vi "main_grid_forming.vi"() -> ()   [LabVIEW 2021]
uses:
  <vilib>/xnet/xnet.llb/XNET Frame CAN.ctl
  <vilib>/xnet/xnet.llb/XNET Frame Type CAN.ctl
  Helper functions/General Purpose/references.ctl
  Helper functions/General Purpose/measurements.ctl
  Helper functions/Time-sync/time_sync/TypeDef/Synch_shift--cluster.ctl
  <vilib>/Platform/TimedLoop/XDataNode/timing_clust.ctl
  <vilib>/Platform/TimedLoop/XDataNode/nitl_modes.ctl
  <vilib>/Platform/TimedLoop/XDataNode/wakeup.ctl
  Helper functions/communication/AFE_froming_Central.ctl
  Helper functions/communication/AFE_froming_Central_Info.ctl
  Helper functions/communication/AFE_froming_Central_Data.ctl
  <vilib>/xnet/xnet.llb/XNET Write (Frame CAN).vi
  <vilib>/xnet/xnet.llb/XNET Read (Frame CAN).vi
  <vilib>/Platform/TimedLoop/XDataNode/XDataNode.xnode
  <vilib>/Platform/TimedLoop/XDataNode/XDNodeRunTimeDep.lvlib
  <userlib>/_OpenG.lib/boolean/boolean.llb/openg_boolean__ogtk.lvlib
panel:
  in  "delta V":dbl format="%#_13g"
  in  "delta f":dbl=0.005800000000000027 format="%#_13g"
  in  "biasQ4":dbl=200.0
  in  "biasQ3":dbl=200.0
  in  "biasQ2":dbl=200.0
  in  "biasQ1":dbl=200.0
  in  "biasV4":dbl
  in  "biasV3":dbl
  in  "biasV2":dbl
  in  "biasV1":dbl=0.6
  out "form":timestamp
  out "follow":timestamp
  out "time_afe":timestamp
  out "start following 1 pre":bool
  out "t_rising":timestamp
  out "t_risingedge":dbl
  out "Synch Monitor":string[][](table)
  in  "Loop Time":u32=125
  out "Error out":errorcluster
  in  "Timeout [ms]":i32=3000
  out "Offset from TR (ns)":dbl
  out "Status Out":T1
  out "CAN OUT":T2[](array[typedef]) {"payload" format="%x"; "timestamp" format="%<%.7X\n%x>T"; "type" items=["CAN Data"=0, "CAN Remote"=1, "CAN Bus Error"=2, "CAN 2.0 Data"=8, "CAN FD Data"=16, "CAN FD+BRS Data"=24, "J1939 Data"=192, "Delay"=224, "Log Trigger"=225, "Start Trigger"=226]; "identifier" format="%x"}
  in  "freq 2":dbl=50.0
  in  "freq 1":dbl=50.0
  in  "Vabs 1":dbl=230.0
  in  "Varg 1":dbl
  in  "Start following 2":bool
  in  "Start following 1":bool
  in  "Vabs 2":dbl=230.0
  in  "Varg 2":dbl
  out "Forming 2":bool
  out "Forming 1":bool
  in  "Start forming 2":bool
  in  "Start forming 1":bool
  out "current time":timestamp
  in  "measurements":T4
  in  "references":T5
  in  "To ACT CH 4":bool
  in  "To ACT CH 3":bool
  in  "To ACT CH 2":bool
  out "Error 4":bool
  out "Fault 4":bool
  out "Error 3":bool
  out "Fault 3":bool
  out "Error 2":bool
  out "Fault 2":bool
  out "State code 4":i32
  out "State code 3":i32
  out "State code 2":i32
  out "State code 1":i32
  out "Error 1":bool
  out "Fault 1":bool
  in  "To ACT CH 1":bool
  in  "main stop":bool
  in  "Vdc4":dbl=750.0
  in  "Qac4":dbl
  in  "Vdc3":dbl=750.0
  in  "Qac3":dbl
  in  "Vdc2":dbl=750.0
  in  "Qac2":dbl
  in  "Emergency 4":bool
  in  "To IN OP  4":bool
  in  "SEND sp 4":bool
  in  "Clear 4":bool
  in  "Shutdwn 4":bool
  in  "Emergency 3":bool
  in  "To IN OP  3":bool
  in  "SEND sp 3":bool
  in  "Clear 3":bool
  in  "Shutdwn 3":bool
  in  "Emergency 2":bool
  in  "To IN OP  2":bool
  in  "SEND sp 2":bool
  in  "Clear 2":bool
  in  "Shutdwn 2":bool
  out "V slider 22":dbl(slide) caption="V-i" max=-10.0 scale=650.0..780.0 scale format="%#_4g"
  out "V slider 21":dbl(slide) caption="V-i" max=-10.0 scale=650.0..780.0 scale format="%#_4g"
  out "V slider 20":dbl(slide) caption="V-i" max=-10.0 scale=650.0..780.0 scale format="%#_4g"
  out "kW":dbl caption="Numeric" format="%#.3g"
  out "?VkVAr":dbl caption="Numeric" format="%.3g"
  out "kW":dbl caption="Numeric" format="%#.3g"
  out "?VkVAr":dbl caption="Numeric" format="%.3g"
  out "kW":dbl caption="Numeric" format="%#.3g"
  out "?VkVAr":dbl caption="Numeric" format="%.3g"
  out "OFF 4":bool
  out "ON 4":bool
  out "Ready 4":bool
  out "OFF 3":bool
  out "ON 3":bool
  out "Ready 3":bool
  out "OFF 2":bool
  out "ON 2":bool
  out "Ready 2":bool
  out "error out":errorcluster
  out "?VkVAr":dbl caption="Numeric" format="%.3g"
  out "kW":dbl caption="Numeric" format="%#.3g"
  out "V slider 19":dbl(slide) caption="V-i" max=-10.0 scale=650.0..780.0 scale format="%#_4g"
  in  "Vdc1":dbl=750.0
  out "OFF 1":bool
  out "ON 1":bool
  out "Ready 1":bool
  out "CAN IN":T2 {"payload" format="%x"; "timestamp" format="%<%.7X\n%x>T"; "type" items=["CAN Data"=0, "CAN Remote"=1, "CAN Bus Error"=2, "CAN 2.0 Data"=8, "CAN FD Data"=16, "CAN FD+BRS Data"=24, "J1939 Data"=192, "Delay"=224, "Log Trigger"=225, "Start Trigger"=226]; "identifier" format="%x"}
  in  "Emergency 1":bool
  in  "Qac1":dbl
  in  "conv":T6
  in  "CAN [ms]":i64=1
  out "CAN with Conv":bool
  out "Measurements":bool
  in  "Shutdwn 1":bool
  in  "Clear 1":bool
  in  "SEND sp 1":bool
  in  "To IN OP 1":bool
  out "logging":bool
  # "Resource agents: AFE 1-4"
  # "package identifiers:\n1xx VSC1 \n2xx VSC2\n3xx VSC3\n4xx VSC4\n\nx0x send from agent to resource\nx02 Power setpoints\nx06 Measurements\nx9 status\n          = [state; error; alarm; OFF; Ready; ON]\n\n \n\nx1x send from resource to agent\nx10 Power measurements\nx11 Measurements\nx12 status\n          = [state; error; alarm; full; precharge; neg; 0; 0]"
  # "B18"
  # "B 22\nB19"
  # "VSC 4"
  # "B17"
  # "B21"
  # "VSC 3"
  # "B16"
  # "B20"
  # "Start-up - Shut down"
  # "VSC 2"
  # "B15"
  # "B19"
  # "Start-up - Shut down"
  # "VSC 1"
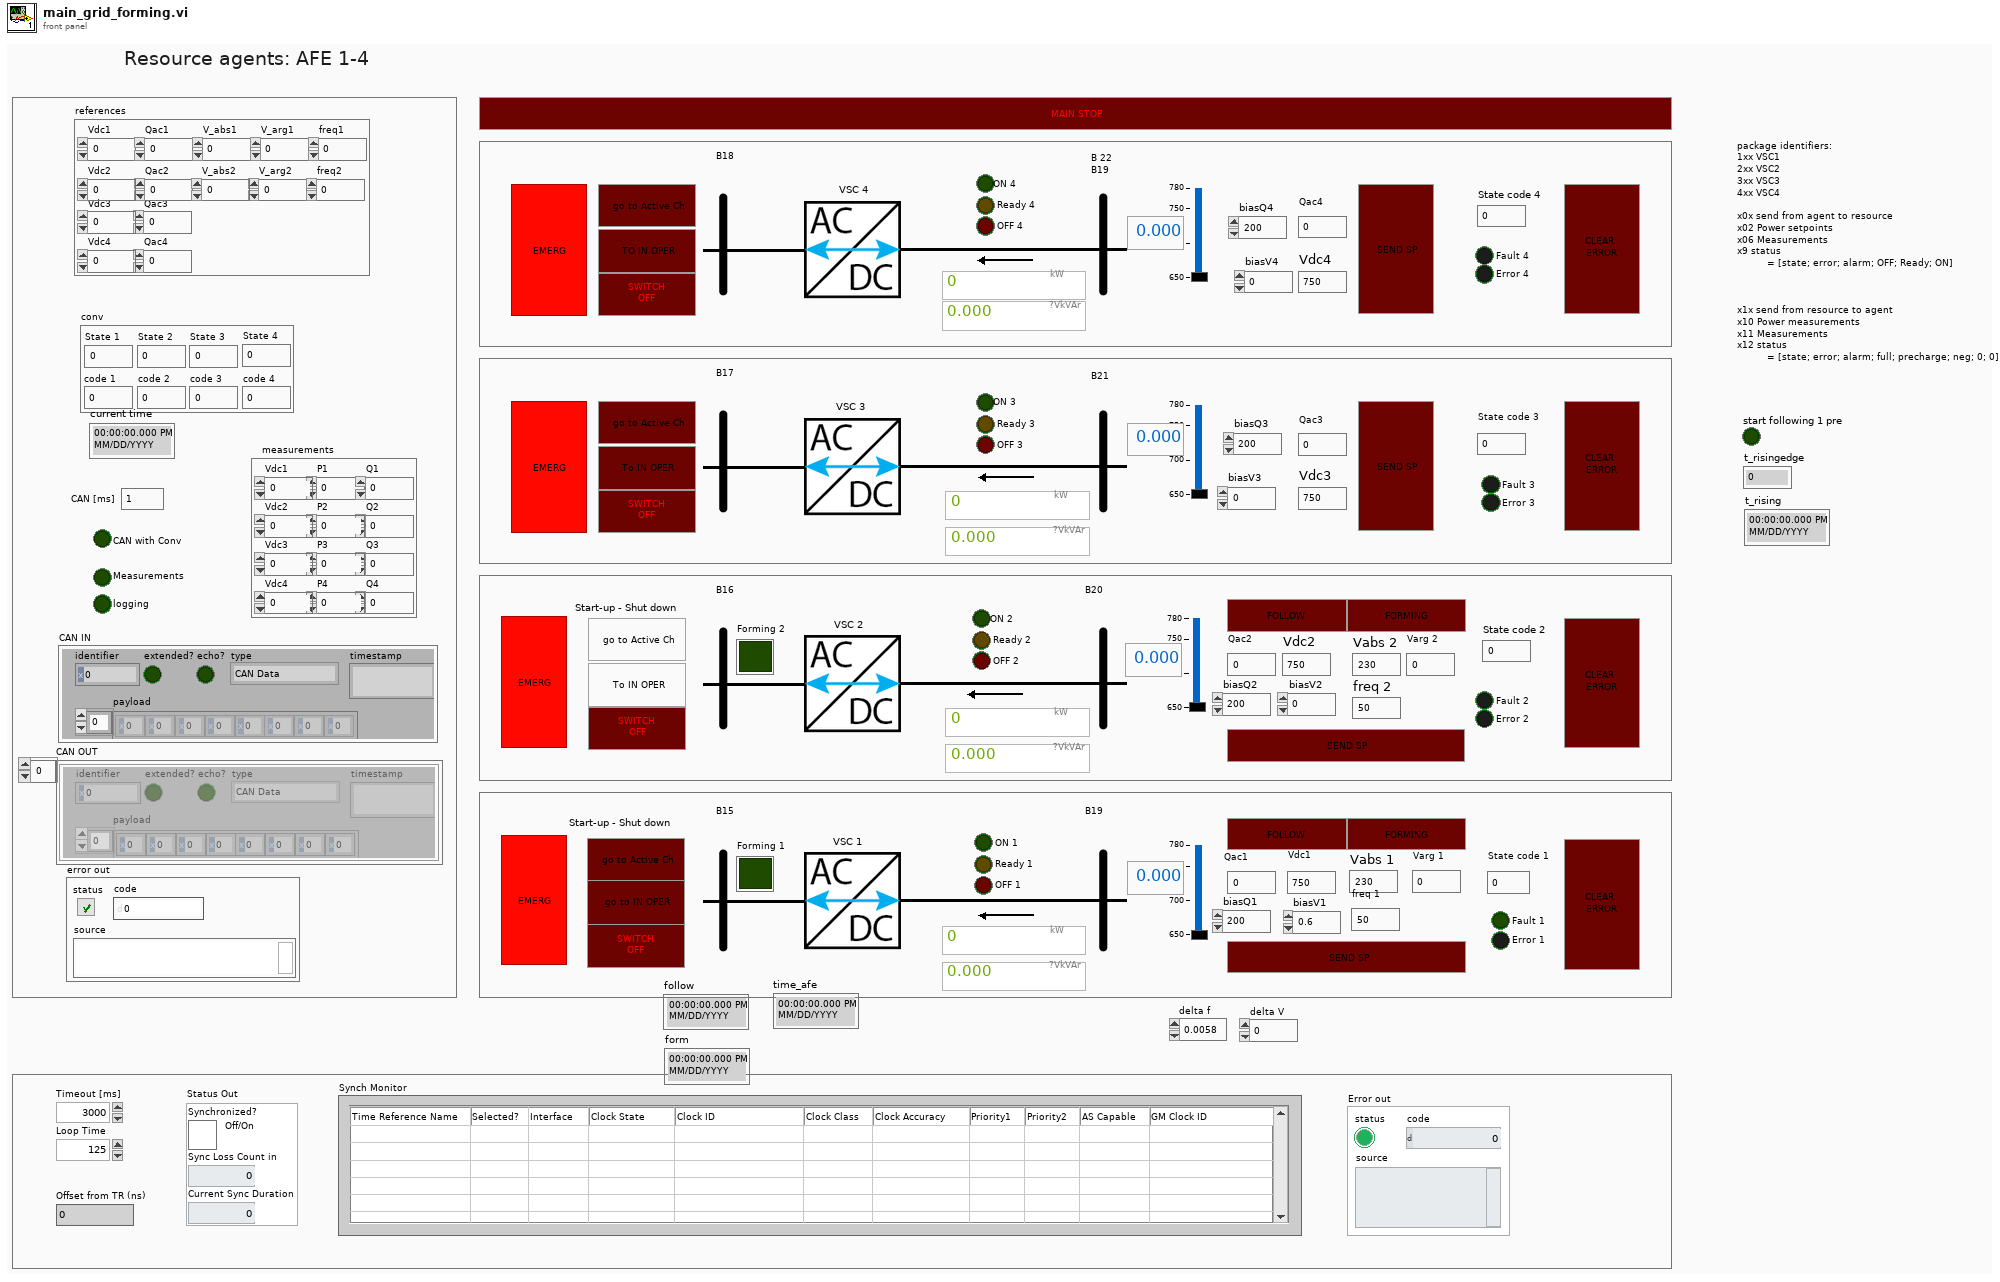
[diagram p1: front panel]
types:
  T1 = typedef "Synch_shift--cluster.ctl" = cluster{"Synchronized?":bool, "Sync Loss Count in":u32, "Current Sync Duration":u32}
  T2 = typedef "XNET Frame CAN.ctl" = cluster{"timestamp":timestamp, "payload":u8[], "identifier":u32, "type":T3, "extended?":bool, "echo?":bool}
  T3 = typedef "XNET Frame Type CAN.ctl" = u8
  T4 = typedef "measurements.ctl" = cluster{"Vdc1":dbl, "P1":dbl, "Vdc2":dbl, "P2":dbl, "Q2":dbl, "Vdc3":dbl, "P3":dbl, "Q3":dbl, "Vdc4":dbl, "P4":dbl, "Q4":dbl, "Q1":dbl}
  T5 = typedef "references.ctl" = cluster{"Vdc1":dbl, "Vdc2":dbl, "Qac2":dbl, "Vdc3":dbl, "Qac3":dbl, "Vdc4":dbl, "Qac4":dbl, "Qac1":dbl, "V_arg2":dbl, "V_abs2":dbl, "V_abs1":dbl, "V_arg1":dbl, "freq1":dbl, "freq2":dbl}
  T6 = cluster{"State 1":dbl, "code 1":dbl, "code 2":dbl, "code 3":dbl, "code 4":dbl, "State 2":dbl, "State 3":dbl, "State 4":dbl}
  T7 = cluster{"Frame In":refnum<k21>, "Frame Out":refnum<k21>}
  T8 = typedef "XDNodeRunTimeDep.lvlib/timing_clust.ctl" = cluster{"Expected End [f-1]":u64, "Actual End [f-1]":u64, "Finished Late? [f-1]":bool, "Expected End [i-1]":u64, "Actual End [i-1]":u64, "Finished Late? [i-1]":bool, "Expected Start [i]":u64, "Actual Start [i]":u64, "Expected Start [f]":u64, "Actual Start [f]":u64, "Source Name":string, "Structure Name":string, "Period":i64, "Deadline":i64, "Offset":i64, "Start":i64, "Priority":i32, "Timeout":i32, "Mode":T9, "Wakeup Reason":T10, "Error":errorcluster, "Source Type":string, "Secondary Source Type":string, "Global End Time":u64, "Global Start Time":u64, "Frame Duration":u64, "Iteration Duration":u64, "Assigned CPU":i32, "I/O Scan Engine Mode":u32}
  T9 = typedef "XDNodeRunTimeDep.lvlib/nitl_modes.ctl" = enum32{"No Change", "Process missed periods, maintain original phase", "Discard missed periods, maintain original phase", "Process missed periods, ignore original phase", "Discard missed periods, ignore original phase"}
  T10 = typedef "XDNodeRunTimeDep.lvlib/wakeup.ctl" = enum32{"Normal", "Aborted", "Asynchronous wakeup", "Timing source error", "Timed loop error", "Timeout"}
  T11 = typedef "AFE_froming_Central.ctl" = cluster{"Info":T12, "Data":T13}
  T12 = typedef "AFE_froming_Central_Info.ctl" = cluster{"Resource":string, "Problem":bool, "Timestamp":dbl}
  T13 = typedef "AFE_froming_Central_Data.ctl" = cluster{"Start forming 1":bool, "Forming/Following":bool[], "Start forming 2":bool, "measurements":cluster{"Vdc1":dbl, "P1":dbl, "Vdc2":dbl, "P2":dbl, "Q2":dbl, "Vdc3":dbl, "P3":dbl, "Q3":dbl, "Vdc4":dbl, "P4":dbl, "Q4":dbl, "Q1":dbl}, "Status":bool[], "references":T5, "Start following 1":bool, "Start following 2":bool}
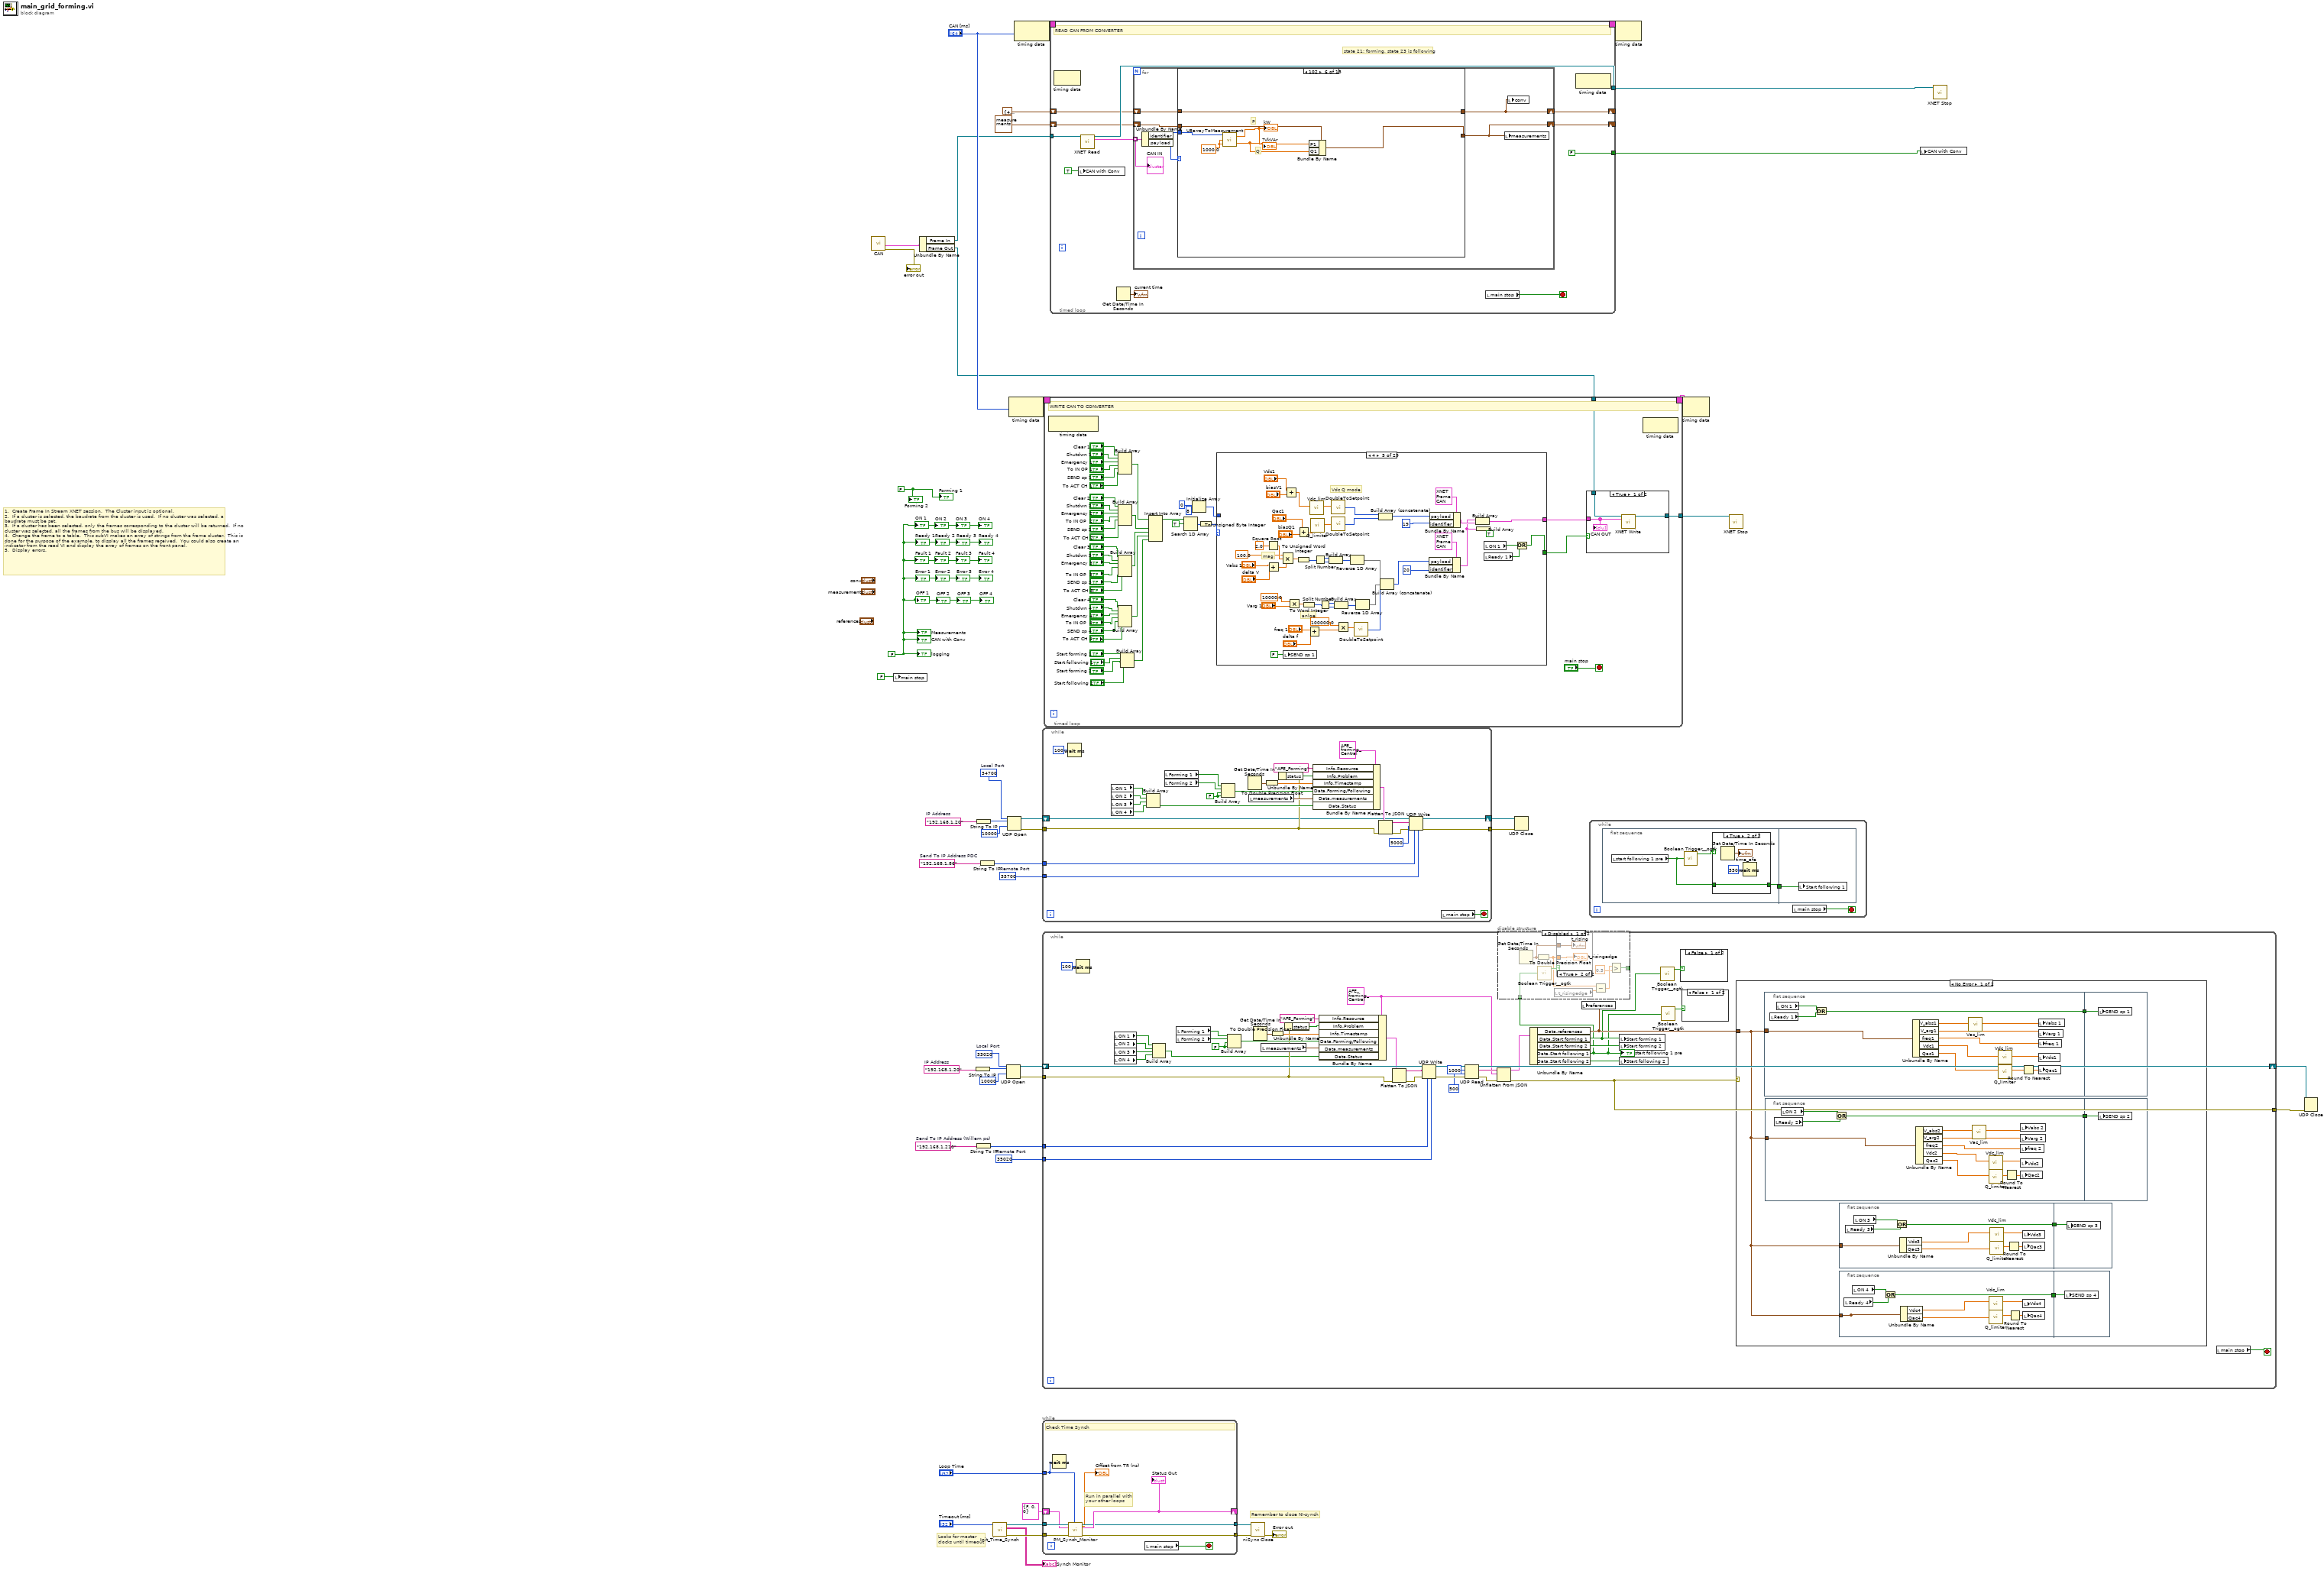
[diagram p0: block diagram]
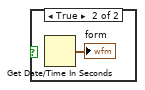
[diagram p3: hidden frame]
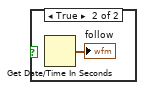
[diagram p4: hidden frame]
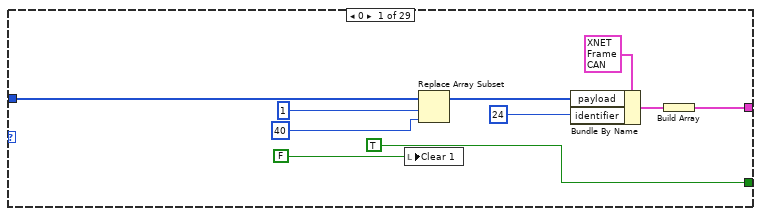
[diagram p9: hidden frame]
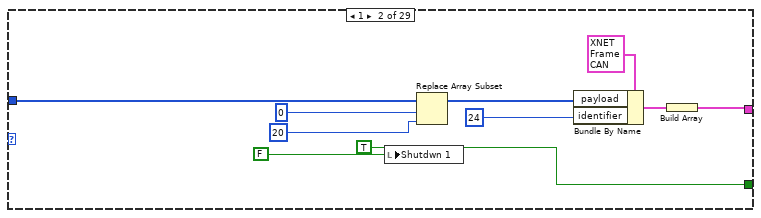
[diagram p10: hidden frame]
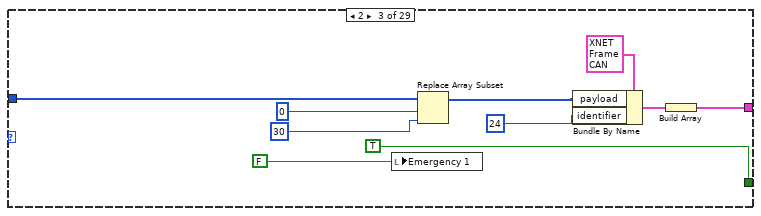
[diagram p11: hidden frame]
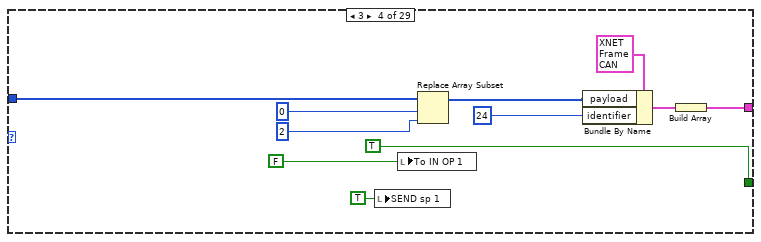
[diagram p12: hidden frame]
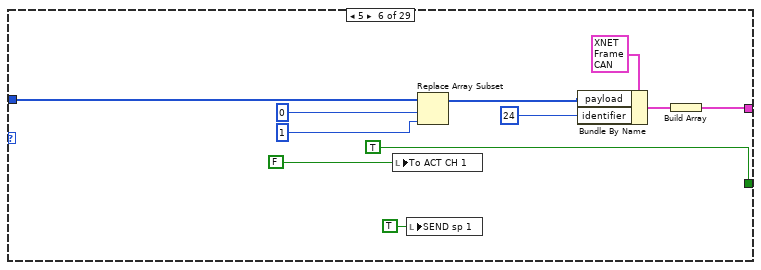
[diagram p13: hidden frame]
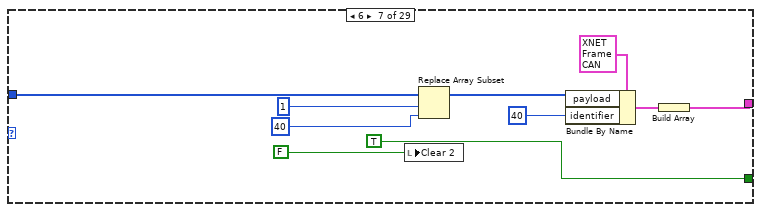
[diagram p14: hidden frame]
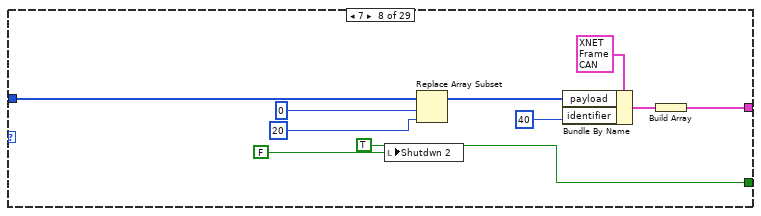
[diagram p15: hidden frame]
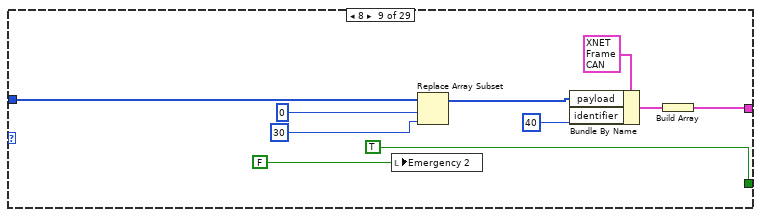
[diagram p16: hidden frame]
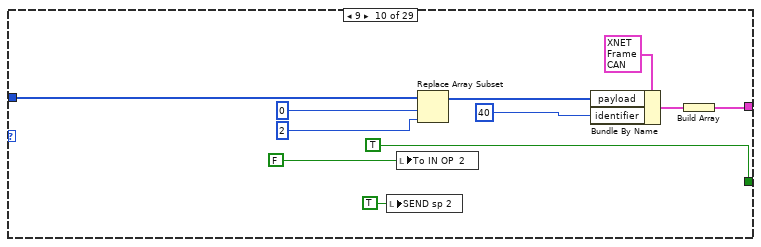
[diagram p17: hidden frame]
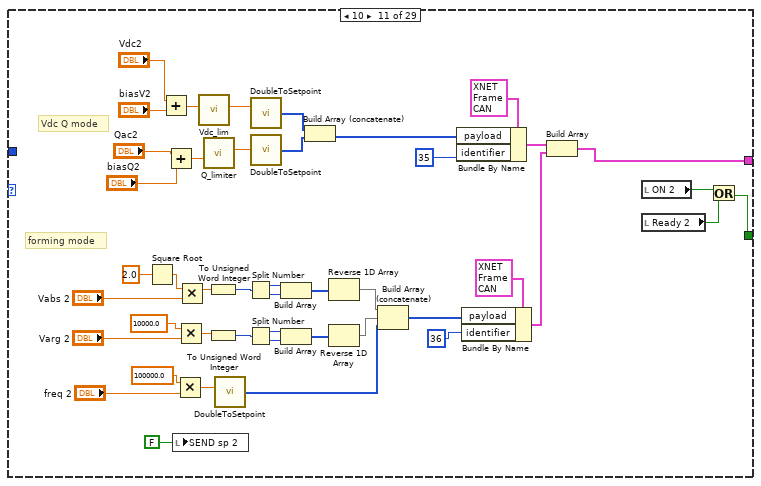
[diagram p18: hidden frame]
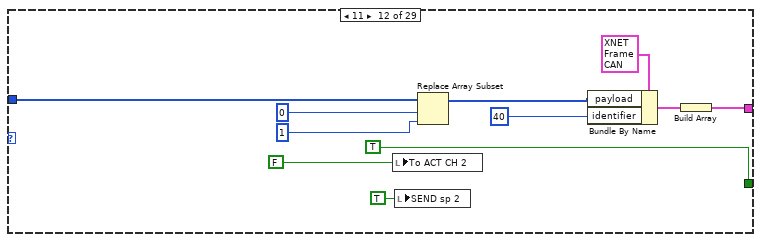
[diagram p19: hidden frame]
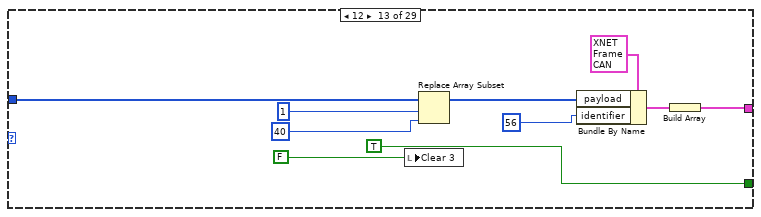
[diagram p20: hidden frame]
diagram:
  w7 = u16 35020  # Remote Port
  w13 = "192.168.1.210"  # Send To IP Address (Willem pc)
  w15 = u16 33020  # Local Port
  w16 = "192.168.1.20"  # IP Address
  w28 = FALSE ("Forming")
  w4 = u16 35700  # Remote Port
  w29 = "192.168.1.86"  # Send To IP Address PDC
  w31 = u16 34700  # Local Port
  w32 = "192.168.1.20"  # IP Address
  w34 = FALSE
  # "Remember to close NI-synch"
  # "Looks for master \nclocks until timeout"
  # "1.  Create Frame In Stream XNET session.  The Cluster input is optional.  \n2.  If a cluster is selected, the baudrate from the cluster is used.  If no cluster was selected, a baudrate must be set.\n3.  If a cluster has been selected, only the frames corresponding to the cluster will be returned.  If no cluster was selected, all the frames from the bus will be displayed.\n4.  Change the frame to a table.  This subVI makes an array of strings from the frame cluster.  This is done for the purpose of the example, to display all the frames received.  You could also create an indicator from the read VI and display the array of frames on the front panel. \n5.  Display errors."
  n1 = call "CAN.vi"() -> ("error out"=→"error out":errorcluster, "CAN"=w36:T7)  [unwired: 10 in]
  n2 = local write "main stop"(FALSE ("main stop")) -> ()
  n3 = Unbundle By Name(w36) -> ("Frame In"=w41:refnum<k21>, "Frame Out"=w44:refnum<k21>)
  n4 = String To IP(1:w16) -> (0:w17:u32)
  n5 = String To IP(1:w32) -> (0:w33:u32)
  n6 = String To IP(1:w13) -> (0:w8:u32)
  n7 = String To IP(1:w29) -> (0:w5:u32)
  n8 = call "Init_Time_Synch.vi"("Timeout [ms]"="Timeout [ms]") -> ("Error out"=w25:errorcluster, "Synch Monitor"=→"Synch Monitor":string[][], "Synch Out"=w23:refnum<k15>)  [unwired: 7 in, 1 out]
  n9 = UDP Open(7:w17, 9:10000 ("timeout ms (25000)"), 11:w15) -> (port=w12:refnum<k16>, 0:w11:errorcluster)  [unwired: 2 in, 1 out]
  n10 = UDP Open(7:w33, 9:10000 ("timeout ms (25000)"), 11:w31) -> (port=w3:refnum<k16>, 0:w2:errorcluster)  [unwired: 2 in, 1 out]
  n11 = node-c288("CAN [ms]") -> (w38:T8)
  n12 = node-c288("CAN [ms]") -> (w43:T8)
  n13 = while {
    tunnel: w11 -> [w66]
    shift-right: [w83] -> w10
    shift-left: w12 -> [w85]
    tunnel: [w86] -> w9
    tunnel: w8 -> [w75]
    tunnel: w7 -> [w79]
    stop <- w88 stop-if-true
    w63 = FALSE ("ON 1")
    w56 = T11 {"Info"={"Resource"="AFE_Forming", "Problem"=FALSE, "Timestamp"=0.0}, "Data"={"Start forming 1"=FALSE, "Forming/Following"=[], "Start forming 2"=FALSE, "measurements"={"Vdc1"=0.0, "P1"=0.0, "Vdc2"=0.0, "P2"=0.0, "Q2"=0.0, "Vdc3"=0.0, "P3"=0.0, "Q3"=0.0, "Vdc4"=0.0, "P4"=0.0, "Q4"=0.0, "Q1"=0.0}, "Status"=[], "references"={"Vdc1"=0.0, "Vdc2"=0.0, "Qac2"=0.0, "Vdc3"=0.0, "Qac3"=0.0, "Vdc4"=0.0, "Qac4"=0.0, "Qac1"=0.0, "V_arg2"=0.0, "V_abs2"=0.0, "V_abs1"=0.0, "V_arg1"=0.0, "freq1"=0.0, "freq2"=0.0}, "Start following 1"=FALSE, "Start following 2"=FALSE}} ("Cluster")
    n14 = Wait (ms)(milliseconds to wait=u32 100) -> ()  [unwired: 1 out]
    n15 = local read "ON 1"() -> (w61:bool)
    n16 = local read "ON 2"() -> (w62:bool)
    n17 = local read "ON 3"() -> (w59:bool)
    n18 = local read "ON 4"() -> (w58:bool)
    n19 = Build Array(w61, w62, w59, w58) -> (w60:bool[])
    n20 = local read "Forming 1"() -> (w65:bool)
    n21 = local read "Forming 2"() -> (w64:bool)
    n22 = Build Array(w65, w64, w63, w63) -> (w72:bool[])
    n23 = Get Date/Time In Seconds() -> (seconds since 1Jan1904=w68:timestamp)
    n24 = local read "measurements"() -> (w57:T4)
    n25 = To Double Precision Float(number=w68) -> (double precision float=w71:dbl)
    n26 = Unbundle By Name(w66) -> ("status"=w67:bool)
    n27 = Bundle By Name(cluster=w56, "Info.Resource"="AFE_Forming", "Info.Problem"=w67, "Info.Timestamp"=w71, "Data.Forming/Following"=w72, "Data.measurements"=w57, "Data.Status"=w60) -> (w69:T11)
    n28 = Flatten To JSON(anything=w69, error in (no error)=w66) -> (JSON string=w74:string, 11:w73:errorcluster)  [unwired: 1 in]
    n29 = UDP Write(address=w75, port or service name=w79, connection ID=w85, data in=w74, 8:w73) -> (error out=w81:errorcluster, 3:w84:refnum<k16>)  [unwired: 1 in]
    n30 = UDP Read(connection ID=w84, max size (548)=1000, timeout ms (25000)=500, 8:w81) -> (data out=w82:string, error out=w78:errorcluster, 3:w83:refnum<k16>)  [unwired: 2 out]
    n31 = Unflatten From JSON(JSON string=w82, type and defaults=w56, error in (no error)=w78) -> (value=w76:T11, error out=w86:errorcluster)  [unwired: 4 in]
    n32 = Unbundle By Name(w76) -> ("Data.references"=w87:T5, "Data.Start forming 1"=w50:bool, "Data.Start forming 2"=w54:bool, "Data.Start following 1"=w49:bool, "Data.Start following 2"=w53:bool)
    "start following 1 pre" <- w49
    n33 = disable-structure shown="Disabled" {
      disable-tunnel: [w95 _] -> _
      disable-tunnel: w49 -> [w93 _]
      frame Disabled {
        n34 = Get Date/Time In Seconds() -> (seconds since 1Jan1904=w94:timestamp)
        n35 = To Double Precision Float(number=w94) -> (double precision float=w96:dbl)
        n36 = call <userlib>:"Boolean Trigger__ogtk.vi"("Boolean Input"=w93) -> ("Rising Edge"=w98:bool)  [unwired: 1 in, 1 out]
        n37 = local read "t_risingedge"() -> (w97:dbl)
        n38 = case shown="True" w98 {
          tunnel: w96 -> [_ w100]
          tunnel: w94 -> [_ w99]
          frame False {
          }
          frame True {
            "t_risingedge" <- w100
            "t_rising" <- w99
          }
        }
        n39 = Subtract(x=w96, y=w97) -> (x-y=w92:dbl)
        n40 = Greater?(x=w92, y=0.5 ("x")) -> (0:w95:bool)
      }
      frame Enabled {
      }
    }
    n41 = local write "references"(w87) -> ()
    n42 = local write "Start forming 1"(w50) -> ()
    n43 = local write "Start forming 2"(w54) -> ()
    n44 = local write "Start following 2"(w53) -> ()
    n45 = call <userlib>:"Boolean Trigger__ogtk.vi"("Boolean Input"=w50) -> ("Rising Edge"=w51:bool)  [unwired: 1 in, 1 out]
    n46 = call <userlib>:"Boolean Trigger__ogtk.vi"("Boolean Input"=w49) -> ("Rising Edge"=w52:bool)  [unwired: 1 in, 1 out]
    n47 = case shown="False" w51 {
      frame False {
      }
      frame True {
        n48 = Get Date/Time In Seconds() -> (seconds since 1Jan1904=→"form":timestamp)
      }
    }
    n49 = case shown="False" w52 {
      frame False {
      }
      frame True {
        n50 = Get Date/Time In Seconds() -> (seconds since 1Jan1904=→"follow":timestamp)
      }
    }
    n51 = case shown="No Error" w86 {
      tunnel: w87 -> [w105 _]
      frame No Error {
        n52 = flat-sequence {
          tunnel: w105 -> [w152]
          tunnel: [w142] -> w103
          tunnel: w103 -> [w153]
          frame #0 {
            n53 = local read "Ready 1"() -> (w144:bool)
            n54 = local read "ON 1"() -> (w143:bool)
            n55 = Or(x=w143, y=w144) -> (x .or. y?=w142:bool)
            n56 = Unbundle By Name(w152) -> ("V_abs1"=w150:dbl, "V_arg1"=w151:dbl, "freq1"=w148:dbl, "Vdc1"=w140:dbl, "Qac1"=w145:dbl)
            n57 = call "Vac_lim.vi"("IN Vdc"=w150) -> ("OUT Vdc"=w149:dbl)  [unwired: 10 in]
            n58 = call "Vdc_lim.vi"("IN Vdc"=w140) -> ("OUT Vdc"=w147:dbl)  [unwired: 10 in]
            n59 = call "Q_limiter.vi"("IN Q"=w145) -> ("OUT Q"=w146:dbl)  [unwired: 10 in]
            n60 = Round To Nearest(number=w146) -> (nearest integer value=w141:dbl)
            n61 = local write "Vabs 1"(w149) -> ()
            n62 = local write "Varg 1"(w151) -> ()
            n63 = local write "freq 1"(w148) -> ()
            n64 = local write "Vdc1"(w147) -> ()
            n65 = local write "Qac1"(w141) -> ()
          }
          frame #1 {
            n66 = local write "SEND sp 1"(w153) -> ()
          }
        }
        n67 = flat-sequence {
          tunnel: w105 -> [w138]
          tunnel: [w128] -> w104
          tunnel: w104 -> [w139]
          frame #0 {
            n68 = local read "Ready 2"() -> (w130:bool)
            n69 = local read "ON 2"() -> (w129:bool)
            n70 = Or(x=w129, y=w130) -> (x .or. y?=w128:bool)
            n71 = Unbundle By Name(w138) -> ("V_abs2"=w137:dbl, "V_arg2"=w135:dbl, "freq2"=w134:dbl, "Vdc2"=w126:dbl, "Qac2"=w131:dbl)
            n72 = call "Vac_lim.vi"("IN Vdc"=w137) -> ("OUT Vdc"=w136:dbl)  [unwired: 10 in]
            n73 = call "Vdc_lim.vi"("IN Vdc"=w126) -> ("OUT Vdc"=w133:dbl)  [unwired: 10 in]
            n74 = call "Q_limiter.vi"("IN Q"=w131) -> ("OUT Q"=w132:dbl)  [unwired: 10 in]
            n75 = Round To Nearest(number=w132) -> (nearest integer value=w127:dbl)
            n76 = local write "Vabs 2"(w136) -> ()
            n77 = local write "Varg 2"(w135) -> ()
            n78 = local write "freq 2"(w134) -> ()
            n79 = local write "Vdc2"(w133) -> ()
            n80 = local write "Qac2"(w127) -> ()
          }
          frame #1 {
            n81 = local write "SEND sp 2"(w139) -> ()
          }
        }
        n82 = flat-sequence {
          tunnel: w105 -> [w124]
          tunnel: [w120] -> w102
          tunnel: w102 -> [w125]
          frame #0 {
            n83 = local read "Ready 3"() -> (w121:bool)
            n84 = local read "ON 3"() -> (w119:bool)
            n85 = Or(x=w119, y=w121) -> (x .or. y?=w120:bool)
            n86 = Unbundle By Name(w124) -> ("Vdc3"=w116:dbl, "Qac3"=w122:dbl)
            n87 = call "Vdc_lim.vi"("IN Vdc"=w116) -> ("OUT Vdc"=w123:dbl)  [unwired: 10 in]
            n88 = call "Q_limiter.vi"("IN Q"=w122) -> ("OUT Q"=w118:dbl)  [unwired: 10 in]
            n89 = Round To Nearest(number=w118) -> (nearest integer value=w117:dbl)
            n90 = local write "Vdc3"(w123) -> ()
            n91 = local write "Qac3"(w117) -> ()
          }
          frame #1 {
            n92 = local write "SEND sp 3"(w125) -> ()
          }
        }
        n93 = flat-sequence {
          tunnel: [w114] -> _
          tunnel: w105 -> [w114]
          tunnel: [w108] -> w101
          tunnel: w101 -> [w115]
          frame #0 {
            n94 = local read "Ready 4"() -> (w110:bool)
            n95 = local read "ON 4"() -> (w109:bool)
            n96 = Or(x=w109, y=w110) -> (x .or. y?=w108:bool)
            n97 = Unbundle By Name(w114) -> ("Vdc4"=w106:dbl, "Qac4"=w111:dbl)
            n98 = call "Vdc_lim.vi"("IN Vdc"=w106) -> ("OUT Vdc"=w113:dbl)  [unwired: 10 in]
            n99 = call "Q_limiter.vi"("IN Q"=w111) -> ("OUT Q"=w112:dbl)  [unwired: 10 in]
            n100 = Round To Nearest(number=w112) -> (nearest integer value=w107:dbl)
            n101 = local write "Vdc4"(w113) -> ()
            n102 = local write "Qac4"(w107) -> ()
          }
          frame #1 {
            n103 = local write "SEND sp 4"(w115) -> ()
          }
        }
      }
      frame Error {
      }
    }
    n104 = local read "main stop"() -> (w88:bool)
  }
  n105 = while {
    tunnel: [w160] -> w6
    tunnel: w5 -> [w158]
    tunnel: w4 -> [w159]
    tunnel: w2 -> [w157]
    shift-right: [w155] -> w1
    shift-left: w3 -> [w156]
    stop <- w154 stop-if-true
    w177 = FALSE ("ON 1")
    n106 = Wait (ms)(milliseconds to wait=u32 100) -> ()  [unwired: 1 out]
    n107 = local read "ON 1"() -> (w170:bool)
    n108 = local read "ON 2"() -> (w169:bool)
    n109 = local read "ON 3"() -> (w171:bool)
    n110 = local read "ON 4"() -> (w172:bool)
    n111 = Build Array(w170, w169, w171, w172) -> (w173:bool[])
    n112 = local read "Forming 1"() -> (w176:bool)
    n113 = local read "Forming 2"() -> (w175:bool)
    n114 = Build Array(w176, w175, w177, w177) -> (w174:bool[])
    n115 = Get Date/Time In Seconds() -> (seconds since 1Jan1904=w165:timestamp)
    n116 = local read "measurements"() -> (w168:T4)
    n117 = To Double Precision Float(number=w165) -> (double precision float=w166:dbl)
    n118 = Unbundle By Name(w157) -> ("status"=w178:bool)
    n119 = Bundle By Name(cluster=T11 {"Info"={"Resource"="AFE_Forming", "Problem"=FALSE, "Timestamp"=0.0}, "Data"={"Start forming 1"=FALSE, "Forming/Following"=[], "Start forming 2"=FALSE, "measurements"={"Vdc1"=0.0, "P1"=0.0, "Vdc2"=0.0, "P2"=0.0, "Q2"=0.0, "Vdc3"=0.0, "P3"=0.0, "Q3"=0.0, "Vdc4"=0.0, "P4"=0.0, "Q4"=0.0, "Q1"=0.0}, "Status"=[], "references"={"Vdc1"=0.0, "Vdc2"=0.0, "Qac2"=0.0, "Vdc3"=0.0, "Qac3"=0.0, "Vdc4"=0.0, "Qac4"=0.0, "Qac1"=0.0, "V_arg2"=0.0, "V_abs2"=0.0, "V_abs1"=0.0, "V_arg1"=0.0, "freq1"=0.0, "freq2"=0.0}, "Start following 1"=FALSE, "Start following 2"=FALSE}} ("Cluster"), "Info.Resource"="AFE_Forming", "Info.Problem"=w178, "Info.Timestamp"=w166, "Data.Forming/Following"=w174, "Data.measurements"=w168, "Data.Status"=w173) -> (w180:T11)
    n120 = Flatten To JSON(anything=w180, error in (no error)=w157) -> (JSON string=w163:string, 11:w164:errorcluster)  [unwired: 1 in]
    n121 = UDP Write(address=w158, port or service name=w159, connection ID=w156, data in=w163, 8:w164, 9:5000 ("timeout ms (25000)")) -> (error out=w160:errorcluster, 3:w155:refnum<k16>)
    n122 = local read "main stop"() -> (w154:bool)
  }
  n123 = while {
    tunnel: w25 -> [w185]
    tunnel: [w186] -> w20
    shift-right: [w187] -> _
    shift-left: T1 {"Synchronized?"=FALSE, "Sync Loss Count in"=0, "Current Sync Duration"=0} ("Status In") -> [w188]
    tunnel: w23 -> [w189]
    tunnel: "Loop Time" -> [w182]
    tunnel: [w184] -> w21
    stop <- w181 stop-if-true
    # "Run in parallel with \nyour other loops"
    # "Check Time Synch"
    n124 = Wait (ms)(milliseconds to wait=w182) -> ()  [unwired: 1 out]
    n125 = call "PM_Synch_Monitor.vi"("Polling Interval"=w182, "error in"=w185, "Status In"=w188, "Synch In"=w189) -> ("error out"=w186:errorcluster, "Status Out"=w187:T1, "Reference out"=w184:refnum<k15>, "Offset from TR (ns)"=→"Offset from TR (ns)":dbl)  [unwired: 3 in, 1 out]
    "Status Out" <- w187
    n126 = local read "main stop"() -> (w181:bool)
  }
  n127 = timed-loop {
    tunnel: w44 -> [w231]
    tunnel: [w230] -> w47
    timing: w38 -> [_]
    timing-out: [_] -> w37
    stop <- "main stop" stop-if-true
    # "WRITE CAN TO CONVERTER"
    n128 = node-c288() -> ()  [unwired: 1 in, 1 out]
    n129 = Build Array("Clear 1", "Shutdwn 1", "Emergency 1", "To IN OP 1", "SEND sp 1", "To ACT CH 1") -> (w206:bool[])
    n130 = Build Array("Clear 2", "Shutdwn 2", "Emergency 2", "To IN OP  2", "SEND sp 2", "To ACT CH 2") -> (w205:bool[])
    n131 = Build Array("Clear 3", "Shutdwn 3", "Emergency 3", "To IN OP  3", "SEND sp 3", "To ACT CH 3") -> (w204:bool[])
    n132 = Build Array("Clear 4", "Shutdwn 4", "Emergency 4", "To IN OP  4", "SEND sp 4", "To ACT CH 4") -> (w203:bool[])
    n133 = Build Array("Start forming 1", "Start following 1", "Start forming 2", "Start following 2") -> (w197:bool[])
    n134 = Insert Into Array(array=w206, new element #1=w205, new element #2=w204, new element #3=w203, new element #4=w197) -> (w202:bool[])  [unwired: 1 in]
    n135 = Search 1D Array(1D array=w202, element=TRUE) -> (index of element=w224:i32)  [unwired: 1 in]
    n136 = Initialize Array(u8 0, 8 ("dimension size")) -> (w232:u8[])
    n137 = To Unsigned Byte Integer(number=w224) -> (unsigned 8bit integer=w228:u8)
    n138 = case shown="4" w228 {
      tunnel: w232 -> [w248 w258 w268 w279 _ w339 w349 w359 w369 w380 _ w435 w445 w455 w465 w476 _ w506 w516 w526 w536 w547 _ w577 w589 w603 w614 w625 w627]
      tunnel: [TRUE TRUE TRUE TRUE w328 TRUE TRUE TRUE TRUE TRUE w422 TRUE TRUE TRUE TRUE TRUE w494 TRUE TRUE TRUE TRUE TRUE w564 TRUE w580 TRUE TRUE TRUE FALSE] -> w195
      tunnel: [w240 w252 w260 w271 w295 w332 w341 w352 w361 w372 w417 w428 w437 w447 w457 w468 w488 w497 w510 w520 w530 w539 w559 w568 w582 w595 w607 w618 w629] -> w194
      frame 0 {
        n139 = local write "Clear 1"(FALSE ("Clear")) -> ()
        n140 = Replace Array Subset(array=w248, new element=u8 40 ("new element/subarray"), index=1) -> (w242:u8[])
        n141 = Bundle By Name(cluster=T2 {"timestamp"=timestamp(0 s since 1904-01-01), "payload"=[], "identifier"=0, "type"=0, "extended?"=FALSE, "echo?"=FALSE} ("CAN frame 3"), "payload"=w242, "identifier"=u32 24) -> (w243:T2)
        n142 = Build Array(w243) -> (w240:T2[])
      }
      frame 1 {
        n143 = local write "Shutdwn 1"(FALSE ("Shutdwn")) -> ()
        n144 = Replace Array Subset(array=w258, new element=u8 20 ("new element/subarray"), index=0) -> (w251:u8[])
        n145 = Bundle By Name(cluster=T2 {"timestamp"=timestamp(0 s since 1904-01-01), "payload"=[], "identifier"=0, "type"=0, "extended?"=FALSE, "echo?"=FALSE} ("CAN frame 3"), "payload"=w251, "identifier"=u32 24) -> (w253:T2)
        n146 = Build Array(w253) -> (w252:T2[])
      }
      frame 2 {
        n147 = local write "Emergency 1"(FALSE ("Idc cmd")) -> ()
        n148 = Replace Array Subset(array=w268, new element=u8 30 ("new element/subarray"), index=0) -> (w262:u8[])
        n149 = Bundle By Name(cluster=T2 {"timestamp"=timestamp(0 s since 1904-01-01), "payload"=[], "identifier"=0, "type"=0, "extended?"=FALSE, "echo?"=FALSE} ("CAN frame 3"), "payload"=w262, "identifier"=u32 24) -> (w263:T2)
        n150 = Build Array(w263) -> (w260:T2[])
      }
      frame 3 {
        n151 = local write "SEND sp 1"(TRUE ("SEND sp 1")) -> ()
        n152 = local write "To IN OP 1"(FALSE ("Idc cmd")) -> ()
        n153 = Replace Array Subset(array=w279, new element=u8 2 ("new element/subarray"), index=0) -> (w272:u8[])
        n154 = Bundle By Name(cluster=T2 {"timestamp"=timestamp(0 s since 1904-01-01), "payload"=[], "identifier"=0, "type"=0, "extended?"=FALSE, "echo?"=FALSE} ("CAN frame 3"), "payload"=w272, "identifier"=u32 24) -> (w274:T2)
        n155 = Build Array(w274) -> (w271:T2[])
      }
      frame 4 {
        (unwired) TRUE
        # "anlge"
        # "mag"
        # "Vdc Q mode"
        n156 = Square Root(x=2.0) -> (sqrt(x)=w294:dbl)
        n157 = Add(x="Vabs 1", y="delta V") -> (x+y=w283:dbl)
        n158 = Compound Arithmetic op=MULTIPLY(100.0 ("value"), w294, w283) -> (w292:dbl)
        n159 = local write "SEND sp 1"(FALSE ("SEND sp")) -> ()
        n160 = Add(x="Vdc1", y="biasV1") -> (x+y=w290:dbl)
        n161 = Multiply(x=10000.0, y="Varg 1") -> (x*y=w304:dbl)
        n162 = To Unsigned Word Integer(number=w292) -> (unsigned 16bit integer=w309:u16)
        n163 = Add(x="Qac1", y="biasQ1") -> (x+y=w286:dbl)
        n164 = To Word Integer(number=w304) -> (16bit integer=w305:i16)
        n165 = Add(x="freq 1", y="delta f") -> (x+y=w285:dbl)
        n166 = call "Vdc_lim.vi"("IN Vdc"=w290) -> ("OUT Vdc"=w320:dbl)  [unwired: 10 in]
        n167 = call "Q_limiter.vi"("IN Q"=w286) -> ("OUT Q"=w319:dbl)  [unwired: 10 in]
        n168 = Split Number(x=w309) -> (hi(x)=w310:u8, lo(x)=w311:u8)
        n169 = Split Number(x=w305) -> (hi(x)=w306:u8, lo(x)=w307:u8)
        n170 = Build Array(w310, w311) -> (w312:u8[])
        n171 = call "DoubleToSetpoint.vi"("Double"=w320) -> ("SP"=w322:u8[])
        n172 = call "DoubleToSetpoint.vi"("Double"=w319) -> ("SP"=w321:u8[])
        n173 = Build Array(w306, w307) -> (w308:u8[])
        n174 = Multiply(x=100000.0, y=w285) -> (x*y=w314:dbl)
        n175 = Reverse 1D Array(array=w312) -> (reversed array=w303:u8[])
        n176 = call "DoubleToSetpoint.vi"("Double"=w314) -> ("SP"=w301:u8[])
        n177 = Reverse 1D Array(array=w308) -> (reversed array=w302:u8[])
        n178 = Build Array (concatenate)(w322, w321) -> (w324:u8[])
        n179 = Build Array (concatenate)(w303, w302, w301) -> (w299:u8[])
        n180 = Bundle By Name(cluster=T2 {"timestamp"=timestamp(0 s since 1904-01-01), "payload"=[], "identifier"=0, "type"=0, "extended?"=FALSE, "echo?"=FALSE} ("CAN frame 3"), "payload"=w299, "identifier"=u32 20) -> (w296:T2)
        n181 = Bundle By Name(cluster=T2 {"timestamp"=timestamp(0 s since 1904-01-01), "payload"=[], "identifier"=0, "type"=0, "extended?"=FALSE, "echo?"=FALSE} ("CAN frame 3"), "payload"=w324, "identifier"=u32 19) -> (w297:T2)
        n182 = Build Array(w296, w297) -> (w295:T2[])
        n183 = Build Array(w296) -> ()  [unwired: 1 out]
        n184 = local read "Ready 1"() -> (w326:bool)
        n185 = local read "ON 1"() -> (w327:bool)
        n186 = Or(x=w327, y=w326) -> (x .or. y?=w328:bool)
      }
      frame 5 {
        n187 = local write "To ACT CH 1"(FALSE ("Idc cmd")) -> ()
        n188 = local write "SEND sp 1"(TRUE ("SEND sp 1")) -> ()
        n189 = Replace Array Subset(array=w339, new element=u8 1 ("new element/subarray"), index=0) -> (w331:u8[])
        n190 = Bundle By Name(cluster=T2 {"timestamp"=timestamp(0 s since 1904-01-01), "payload"=[], "identifier"=0, "type"=0, "extended?"=FALSE, "echo?"=FALSE} ("CAN frame 3"), "payload"=w331, "identifier"=u32 24) -> (w333:T2)
        n191 = Build Array(w333) -> (w332:T2[])
      }
      frame 6 {
        n192 = local write "Clear 2"(FALSE ("Clear")) -> ()
        n193 = Replace Array Subset(array=w349, new element=u8 40 ("new element/subarray"), index=1) -> (w343:u8[])
        n194 = Bundle By Name(cluster=T2 {"timestamp"=timestamp(0 s since 1904-01-01), "payload"=[], "identifier"=0, "type"=0, "extended?"=FALSE, "echo?"=FALSE} ("CAN frame 3"), "payload"=w343, "identifier"=u32 40) -> (w344:T2)
        n195 = Build Array(w344) -> (w341:T2[])
      }
      frame 7 {
        n196 = local write "Shutdwn 2"(FALSE ("Shutdwn")) -> ()
        n197 = Replace Array Subset(array=w359, new element=u8 20 ("new element/subarray"), index=0) -> (w353:u8[])
        n198 = Bundle By Name(cluster=T2 {"timestamp"=timestamp(0 s since 1904-01-01), "payload"=[], "identifier"=0, "type"=0, "extended?"=FALSE, "echo?"=FALSE} ("CAN frame 3"), "payload"=w353, "identifier"=u32 40) -> (w354:T2)
        n199 = Build Array(w354) -> (w352:T2[])
      }
      frame 8 {
        n200 = local write "Emergency 2"(FALSE ("Idc cmd")) -> ()
        n201 = Replace Array Subset(array=w369, new element=u8 30 ("new element/subarray"), index=0) -> (w363:u8[])
        n202 = Bundle By Name(cluster=T2 {"timestamp"=timestamp(0 s since 1904-01-01), "payload"=[], "identifier"=0, "type"=0, "extended?"=FALSE, "echo?"=FALSE} ("CAN frame 3"), "payload"=w363, "identifier"=u32 40) -> (w364:T2)
        n203 = Build Array(w364) -> (w361:T2[])
      }
      frame 9 {
        n204 = local write "SEND sp 2"(TRUE ("SEND sp 2")) -> ()
        n205 = local write "To IN OP  2"(FALSE ("Idc cmd")) -> ()
        n206 = Replace Array Subset(array=w380, new element=u8 2 ("new element/subarray"), index=0) -> (w374:u8[])
        n207 = Bundle By Name(cluster=T2 {"timestamp"=timestamp(0 s since 1904-01-01), "payload"=[], "identifier"=0, "type"=0, "extended?"=FALSE, "echo?"=FALSE} ("CAN frame 3"), "payload"=w374, "identifier"=u32 40) -> (w375:T2)
        n208 = Build Array(w375) -> (w372:T2[])
      }
      frame 10 {
        # "forming mode"
        # "Vdc Q mode"
        n209 = Square Root(x=2.0) -> (sqrt(x)=w409:dbl)
        n210 = Add(x="Vdc2", y="biasV2") -> (x+y=w387:dbl)
        n211 = Add(x="Qac2", y="biasQ2") -> (x+y=w382:dbl)
        n212 = local write "SEND sp 2"(FALSE ("SEND sp")) -> ()
        n213 = Multiply(x=100000.0, y="freq 2") -> (x*y=w407:dbl)
        n214 = Multiply(x=10000.0, y="Varg 2") -> (x*y=w397:dbl)
        n215 = Multiply(x=w409, y="Vabs 2") -> (x*y=w396:dbl)
        n216 = call "Vdc_lim.vi"("IN Vdc"=w387) -> ("OUT Vdc"=w414:dbl)  [unwired: 10 in]
        n217 = call "Q_limiter.vi"("IN Q"=w382) -> ("OUT Q"=w413:dbl)  [unwired: 10 in]
        n218 = To Unsigned Word Integer(number=w396) -> (unsigned 16bit integer=w402:u16)
        n219 = To Unsigned Word Integer(number=w397) -> (unsigned 16bit integer=w398:u16)
        n220 = call "DoubleToSetpoint.vi"("Double"=w407) -> ("SP"=w393:u8[])
        n221 = Split Number(x=w402) -> (hi(x)=w403:u8, lo(x)=w404:u8)
        n222 = Split Number(x=w398) -> (hi(x)=w399:u8, lo(x)=w400:u8)
        n223 = call "DoubleToSetpoint.vi"("Double"=w414) -> ("SP"=w416:u8[])
        n224 = call "DoubleToSetpoint.vi"("Double"=w413) -> ("SP"=w415:u8[])
        n225 = Build Array(w403, w404) -> (w405:u8[])
        n226 = Build Array(w399, w400) -> (w401:u8[])
        n227 = Build Array (concatenate)(w416, w415) -> (w419:u8[])
        n228 = Reverse 1D Array(array=w405) -> (reversed array=w395:u8[])
        n229 = Reverse 1D Array(array=w401) -> (reversed array=w394:u8[])
        n230 = Build Array (concatenate)(w395, w394, w393) -> (w389:u8[])
        n231 = Bundle By Name(cluster=T2 {"timestamp"=timestamp(0 s since 1904-01-01), "payload"=[], "identifier"=0, "type"=0, "extended?"=FALSE, "echo?"=FALSE} ("CAN frame 3"), "payload"=w419, "identifier"=u32 35) -> (w420:T2)
        n232 = Bundle By Name(cluster=T2 {"timestamp"=timestamp(0 s since 1904-01-01), "payload"=[], "identifier"=0, "type"=0, "extended?"=FALSE, "echo?"=FALSE} ("CAN frame 3"), "payload"=w389, "identifier"=u32 36) -> (w411:T2)
        n233 = Build Array(w420, w411) -> (w417:T2[])
        n234 = local read "ON 2"() -> (w423:bool)
        n235 = local read "Ready 2"() -> (w424:bool)
        n236 = Or(x=w423, y=w424) -> (x .or. y?=w422:bool)
      }
      frame 11 {
        n237 = local write "To ACT CH 2"(FALSE ("Idc cmd")) -> ()
        n238 = local write "SEND sp 2"(TRUE ("SEND sp 2")) -> ()
        n239 = Replace Array Subset(array=w435, new element=u8 1 ("new element/subarray"), index=0) -> (w427:u8[])
        n240 = Bundle By Name(cluster=T2 {"timestamp"=timestamp(0 s since 1904-01-01), "payload"=[], "identifier"=0, "type"=0, "extended?"=FALSE, "echo?"=FALSE} ("CAN frame 3"), "payload"=w427, "identifier"=u32 40) -> (w429:T2)
        n241 = Build Array(w429) -> (w428:T2[])
      }
      frame 12 {
        n242 = local write "Clear 3"(FALSE ("Clear")) -> ()
        n243 = Replace Array Subset(array=w445, new element=u8 40 ("new element/subarray"), index=1) -> (w439:u8[])
        n244 = Bundle By Name(cluster=T2 {"timestamp"=timestamp(0 s since 1904-01-01), "payload"=[], "identifier"=0, "type"=0, "extended?"=FALSE, "echo?"=FALSE} ("CAN frame 3"), "payload"=w439, "identifier"=u32 56) -> (w440:T2)
        n245 = Build Array(w440) -> (w437:T2[])
      }
      frame 13 {
        n246 = local write "Shutdwn 3"(FALSE ("Shutdwn")) -> ()
        n247 = Replace Array Subset(array=w455, new element=u8 20 ("new element/subarray"), index=0) -> (w449:u8[])
        n248 = Bundle By Name(cluster=T2 {"timestamp"=timestamp(0 s since 1904-01-01), "payload"=[], "identifier"=0, "type"=0, "extended?"=FALSE, "echo?"=FALSE} ("CAN frame 3"), "payload"=w449, "identifier"=u32 56) -> (w450:T2)
        n249 = Build Array(w450) -> (w447:T2[])
      }
      frame 14 {
        n250 = local write "Emergency 3"(FALSE ("Idc cmd")) -> ()
        n251 = Replace Array Subset(array=w465, new element=u8 30 ("new element/subarray"), index=0) -> (w459:u8[])
        n252 = Bundle By Name(cluster=T2 {"timestamp"=timestamp(0 s since 1904-01-01), "payload"=[], "identifier"=0, "type"=0, "extended?"=FALSE, "echo?"=FALSE} ("CAN frame 3"), "payload"=w459, "identifier"=u32 56) -> (w460:T2)
        n253 = Build Array(w460) -> (w457:T2[])
      }
      frame 15 {
        n254 = local write "SEND sp 3"(TRUE ("SEND sp 3")) -> ()
        n255 = local write "To IN OP  3"(FALSE ("Idc cmd")) -> ()
        n256 = Replace Array Subset(array=w476, new element=u8 2 ("new element/subarray"), index=0) -> (w470:u8[])
        n257 = Bundle By Name(cluster=T2 {"timestamp"=timestamp(0 s since 1904-01-01), "payload"=[], "identifier"=0, "type"=0, "extended?"=FALSE, "echo?"=FALSE} ("CAN frame 3"), "payload"=w470, "identifier"=u32 56) -> (w471:T2)
        n258 = Build Array(w471) -> (w468:T2[])
      }
      frame 16 {
        # "Vdc Q mode"
        n259 = local write "SEND sp 3"(FALSE ("SEND sp")) -> ()
        n260 = Add(x="Vdc3", y="biasV3") -> (x+y=w482:dbl)
        n261 = Add(x="Qac3", y="biasQ3") -> (x+y=w478:dbl)
        n262 = call "Vdc_lim.vi"("IN Vdc"=w482) -> ("OUT Vdc"=w485:dbl)  [unwired: 10 in]
        n263 = call "Q_limiter.vi"("IN Q"=w478) -> ("OUT Q"=w484:dbl)  [unwired: 10 in]
        n264 = call "DoubleToSetpoint.vi"("Double"=w485) -> ("SP"=w487:u8[])
        n265 = call "DoubleToSetpoint.vi"("Double"=w484) -> ("SP"=w486:u8[])
        n266 = Build Array (concatenate)(w487, w486) -> (w490:u8[])
        n267 = local read "ON 3"() -> (w495:bool)
        n268 = local read "Ready 3"() -> (w493:bool)
        n269 = Or(x=w495, y=w493) -> (x .or. y?=w494:bool)
        n270 = Bundle By Name(cluster=T2 {"timestamp"=timestamp(0 s since 1904-01-01), "payload"=[], "identifier"=0, "type"=0, "extended?"=FALSE, "echo?"=FALSE} ("CAN frame 3"), "payload"=w490, "identifier"=u32 51) -> (w491:T2)
        n271 = Build Array(w491) -> (w488:T2[])
      }
      frame 17 {
        n272 = local write "To ACT CH 3"(FALSE ("Idc cmd")) -> ()
        n273 = local write "SEND sp 3"(TRUE ("SEND sp 3")) -> ()
        n274 = Replace Array Subset(array=w506, new element=u8 1 ("new element/subarray"), index=0) -> (w499:u8[])
        n275 = Bundle By Name(cluster=T2 {"timestamp"=timestamp(0 s since 1904-01-01), "payload"=[], "identifier"=0, "type"=0, "extended?"=FALSE, "echo?"=FALSE} ("CAN frame 3"), "payload"=w499, "identifier"=u32 56) -> (w500:T2)
        n276 = Build Array(w500) -> (w497:T2[])
      }
      frame 18 {
        n277 = local write "Clear 4"(FALSE ("Clear")) -> ()
        n278 = Replace Array Subset(array=w516, new element=u8 40 ("new element/subarray"), index=1) -> (w509:u8[])
        n279 = Bundle By Name(cluster=T2 {"timestamp"=timestamp(0 s since 1904-01-01), "payload"=[], "identifier"=0, "type"=0, "extended?"=FALSE, "echo?"=FALSE} ("CAN frame 3"), "payload"=w509, "identifier"=u32 72) -> (w511:T2)
        n280 = Build Array(w511) -> (w510:T2[])
      }
      frame 19 {
        n281 = local write "Shutdwn 4"(FALSE ("Shutdwn")) -> ()
        n282 = Replace Array Subset(array=w526, new element=u8 20 ("new element/subarray"), index=0) -> (w519:u8[])
        n283 = Bundle By Name(cluster=T2 {"timestamp"=timestamp(0 s since 1904-01-01), "payload"=[], "identifier"=0, "type"=0, "extended?"=FALSE, "echo?"=FALSE} ("CAN frame 3"), "payload"=w519, "identifier"=u32 72) -> (w521:T2)
        n284 = Build Array(w521) -> (w520:T2[])
      }
      frame 20 {
        n285 = local write "Emergency 4"(FALSE ("Idc cmd")) -> ()
        n286 = Replace Array Subset(array=w536, new element=u8 30 ("new element/subarray"), index=0) -> (w529:u8[])
        n287 = Bundle By Name(cluster=T2 {"timestamp"=timestamp(0 s since 1904-01-01), "payload"=[], "identifier"=0, "type"=0, "extended?"=FALSE, "echo?"=FALSE} ("CAN frame 3"), "payload"=w529, "identifier"=u32 72) -> (w531:T2)
        n288 = Build Array(w531) -> (w530:T2[])
      }
      frame 21 {
        n289 = local write "SEND sp 4"(TRUE ("SEND sp 4")) -> ()
        n290 = local write "To IN OP  4"(FALSE ("Idc cmd")) -> ()
        n291 = Replace Array Subset(array=w547, new element=u8 2 ("new element/subarray"), index=0) -> (w541:u8[])
        n292 = Bundle By Name(cluster=T2 {"timestamp"=timestamp(0 s since 1904-01-01), "payload"=[], "identifier"=0, "type"=0, "extended?"=FALSE, "echo?"=FALSE} ("CAN frame 3"), "payload"=w541, "identifier"=u32 72) -> (w542:T2)
        n293 = Build Array(w542) -> (w539:T2[])
      }
      frame 22 {
        # "Vdc Q mode"
        n294 = Add(x="Qac4", y="biasQ4") -> (x+y=w549:dbl)
        n295 = local write "SEND sp 4"(FALSE ("SEND sp")) -> ()
        n296 = Add(x="Vdc4", y="biasV4") -> (x+y=w553:dbl)
        n297 = call "Q_limiter.vi"("IN Q"=w549) -> ("OUT Q"=w555:dbl)  [unwired: 10 in]
        n298 = call "Vdc_lim.vi"("IN Vdc"=w553) -> ("OUT Vdc"=w556:dbl)  [unwired: 10 in]
        n299 = call "DoubleToSetpoint.vi"("Double"=w556) -> ("SP"=w558:u8[])
        n300 = call "DoubleToSetpoint.vi"("Double"=w555) -> ("SP"=w557:u8[])
        n301 = Build Array (concatenate)(w558, w557) -> (w561:u8[])
        n302 = local read "ON 4"() -> (w565:bool)
        n303 = local read "Ready 4"() -> (w566:bool)
        n304 = Or(x=w565, y=w566) -> (x .or. y?=w564:bool)
        n305 = Bundle By Name(cluster=T2 {"timestamp"=timestamp(0 s since 1904-01-01), "payload"=[], "identifier"=0, "type"=0, "extended?"=FALSE, "echo?"=FALSE} ("CAN frame 3"), "payload"=w561, "identifier"=u32 67) -> (w562:T2)
        n306 = Build Array(w562) -> (w559:T2[])
      }
      frame 23 {
        n307 = local write "To ACT CH 4"(FALSE ("Idc cmd")) -> ()
        n308 = local write "SEND sp 4"(TRUE ("SEND sp 4")) -> ()
        n309 = Replace Array Subset(array=w577, new element=u8 1 ("new element/subarray"), index=0) -> (w570:u8[])
        n310 = Bundle By Name(cluster=T2 {"timestamp"=timestamp(0 s since 1904-01-01), "payload"=[], "identifier"=0, "type"=0, "extended?"=FALSE, "echo?"=FALSE} ("CAN frame 3"), "payload"=w570, "identifier"=u32 72) -> (w571:T2)
        n311 = Build Array(w571) -> (w568:T2[])
      }
      frame 24 {
        # "it take on average 500ms to close the switch\n-> therefore, we wait 200ms so the converter is only following in grid connected mode for 300ms\n-> this guarentees a more smooth stransition"
        # "start forming 1"
        n312 = local write "Start forming 1"(FALSE ("Start following 1")) -> ()
        n313 = local write "SEND sp 1"(TRUE ("SEND sp 1")) -> ()
        n314 = Replace Array Subset(array=w589, new element=u8 3 ("new element/subarray"), index=0) -> (w584:u8[])
        n315 = flat-sequence {
          tunnel: [TRUE] -> w579
          tunnel: [w593] -> w580
          tunnel: w579 -> [w593]
          frame #0 {
          }
          frame #1 {
            # "40"
            n316 = Wait (ms)(milliseconds to wait=u32 80) -> ()  [unwired: 1 out]
          }
        }
        n317 = Bundle By Name(cluster=T2 {"timestamp"=timestamp(0 s since 1904-01-01), "payload"=[], "identifier"=0, "type"=0, "extended?"=FALSE, "echo?"=FALSE} ("CAN frame 3"), "payload"=w584, "identifier"=u32 24) -> (w585:T2)
        n318 = Build Array(w585) -> (w582:T2[])
      }
      frame 25 {
        # "it take on average 140ms to open the switch\n-> to be sure the grid is connected before we stors following, we add a 300ms delay\n-> the converter can easily sustain 160ms in forming mode when grid connected"
        # "start following 1"
        n319 = local write "Start following 1"(FALSE ("Start forming 1")) -> ()
        n320 = local write "SEND sp 1"(TRUE ("SEND sp 1")) -> ()
        n321 = Replace Array Subset(array=w603, new element=u8 2 ("new element/subarray"), index=0) -> (w597:u8[])
        n322 = Bundle By Name(cluster=T2 {"timestamp"=timestamp(0 s since 1904-01-01), "payload"=[], "identifier"=0, "type"=0, "extended?"=FALSE, "echo?"=FALSE} ("CAN frame 3"), "payload"=w597, "identifier"=u32 24) -> (w598:T2)
        n323 = Build Array(w598) -> (w595:T2[])
      }
      frame 26 {
        # "start forming 2"
        n324 = local write "SEND sp 2"(TRUE ("SEND sp 2")) -> ()
        n325 = local write "Start forming 2"(FALSE ("Start following 1")) -> ()
        n326 = Replace Array Subset(array=w614, new element=u8 3 ("new element/subarray"), index=0) -> (w605:u8[])
        n327 = Bundle By Name(cluster=T2 {"timestamp"=timestamp(0 s since 1904-01-01), "payload"=[], "identifier"=0, "type"=0, "extended?"=FALSE, "echo?"=FALSE} ("CAN frame 3"), "payload"=w605, "identifier"=u32 40) -> (w608:T2)
        n328 = Build Array(w608) -> (w607:T2[])
      }
      frame 27 {
        # "start following 2"
        n329 = local write "Start following 2"(FALSE ("Start forming 1")) -> ()
        n330 = local write "SEND sp 2"(TRUE ("SEND sp 2")) -> ()
        n331 = Replace Array Subset(array=w625, new element=u8 2 ("new element/subarray"), index=0) -> (w616:u8[])
        n332 = Bundle By Name(cluster=T2 {"timestamp"=timestamp(0 s since 1904-01-01), "payload"=[], "identifier"=0, "type"=0, "extended?"=FALSE, "echo?"=FALSE} ("CAN frame 3"), "payload"=w616, "identifier"=u32 40) -> (w619:T2)
        n333 = Build Array(w619) -> (w618:T2[])
      }
      frame 99, Default {
        n334 = Bundle By Name(cluster=T2 {"timestamp"=timestamp(0 s since 1904-01-01), "payload"=[], "identifier"=0, "type"=0, "extended?"=FALSE, "echo?"=FALSE} ("CAN frame 3"), "payload"=w627, "identifier"=u32 18) -> (w630:T2)
        n335 = Build Array(w630) -> (w629:T2[])
      }
    }
    n336 = case shown="True" w195 {
      tunnel: w194 -> [w237 _]
      tunnel: w231 -> [w239 _]
      tunnel: [w238 _] -> w230
      frame True {
        n337 = call-poly <vilib>:"XNET Write.vi"("session in"=w239, "data"=w237) -> ("session out"=w238:refnum<k21>)  [unwired: 12 in, 1 out]
        "CAN OUT" <- w237
      }
      frame False {
      }
    }
    n338 = node-c288() -> ()  [unwired: 1 in, 1 out]
  }
  n339 = timed-loop {
    timing: w43 -> [_]
    timing-out: [_] -> w42
    tunnel: w41 -> [w636]
    tunnel: [w642] -> w48
    shift-right: [w637] -> _
    shift-left: T6 {"State 1"=4.0, "code 1"=0.0, "code 2"=0.0, "code 3"=0.0, "code 4"=0.0, "State 2"=4.0, "State 3"=4.0, "State 4"=4.0} ("Conv 2") -> [w641]
    tunnel: [FALSE ("stop CAN")] -> w45
    shift-right: [w634] -> _
    shift-left: T4 {"Vdc1"=0.0, "P1"=0.0, "Vdc2"=0.0, "P2"=0.0, "Q2"=0.0, "Vdc3"=0.0, "P3"=0.0, "Q3"=0.0, "Vdc4"=0.0, "P4"=0.0, "Q4"=0.0, "Q1"=0.0} ("measurements 2") -> [w635]
    stop <- w640 stop-if-true
    # "state 21: forming, state 23 is following"
    # "READ CAN FROM CONVERTER"
    n340 = node-c288() -> ()  [unwired: 1 in, 1 out]
    n341 = local write "CAN with Conv"(TRUE) -> ()
    n342 = call-poly <vilib>:"XNET Read.vi"("session in"=w636) -> ("session out"=w642:refnum<k21>, "data"=w643:T2[])  [unwired: 11 in, 2 out]
    n343 = Get Date/Time In Seconds() -> (seconds since 1Jan1904=→"current time":timestamp)
    n344 = for {
      tunnel: w643 -> [w648] mode=indexing
      shift-right: [w646] -> w637
      shift-left: w641 -> [w647]
      shift-right: [w644] -> w634
      shift-left: w635 -> [w645]
      n345 = Unbundle By Name(w648) -> ("identifier"=w650:u32, "payload"=w649:u8[])
      n346 = case shown="102" w650 {
        tunnel: w649 -> [_ w657 w691 w716 w741 w768 w775 w782 w789 w794 w802 w810 w818]
        tunnel: w647 -> [w652 w665 w699 w724 w749 w766 w773 w780 w787 w792 w798 w807 w815]
        tunnel: [w652 w664 w698 w723 w748 w766 w773 w780 w787 w792 w798 w807 w815] -> w646
        tunnel: w645 -> [w651 w654 w688 w713 w739 w764 w769 w776 w783 w790 w797 w806 w813]
        tunnel: [w651 w655 w689 w714 w740 w765 w770 w777 w784 w791 w796 w805 w814] -> w644
        frame 0, Default {
        }
        frame 25 {
          w653 = 1.0 ("factor 1")
          n347 = Index Array(array=w657, index=0) -> (element=w658:u8)
          n348 = call "U8arrayToMeasurement.vi"("factor 2"=w653, "factor 1"=w653, "payload"=w657) -> ("Meas 2"=w656:dbl)  [unwired: 1 out]
          "V slider 19" <- w656
          n349 = Index Array(array=w657, index=1) -> (element=w661:u8)
          n350 = Index Array(array=w657, index=2) -> (element=w660:u8)
          n351 = Join Numbers(hi=w661, lo=w660) -> ((hi.lo)=w659:u16)
          "State code 1" <- w659
          n352 = Bundle By Name(cluster=w654, "Vdc1"=w656) -> (w655:T4)
          n353 = case shown="5" w658 {
            frame 5 {
              w668 = FALSE ("Fault 1")
              n354 = local write "Forming 1"(FALSE ("Forming 1")) -> ()
              n355 = local write "Fault 1"(TRUE ("Fault 1")) -> ()
              n356 = local write "Error 1"(w668) -> ()
              n357 = local write "OFF 1"(w668) -> ()
              n358 = local write "Ready 1"(w668) -> ()
              n359 = local write "ON 1"(w668) -> ()
            }
            frame 6 {
              w672 = FALSE ("Fault 1")
              n360 = local write "Fault 1"(w672) -> ()
              n361 = local write "Error 1"(w672) -> ()
              n362 = local write "OFF 1"(w672) -> ()
              n363 = local write "Ready 1"(w672) -> ()
              n364 = local write "ON 1"(TRUE ("Fault 1")) -> ()
              n365 = local write "Forming 1"(TRUE ("Forming 1")) -> ()
            }
            frame 1 {
              w674 = FALSE ("Fault 1")
              n366 = local write "Forming 1"(FALSE ("Forming 1")) -> ()
              n367 = local write "Fault 1"(w674) -> ()
              n368 = local write "Error 1"(TRUE ("Error 1")) -> ()
              n369 = local write "OFF 1"(w674) -> ()
              n370 = local write "Ready 1"(w674) -> ()
              n371 = local write "ON 1"(w674) -> ()
            }
            frame 2 {
              w678 = FALSE ("Fault 1")
              n372 = local write "Forming 1"(FALSE ("Forming 1")) -> ()
              n373 = local write "Fault 1"(w678) -> ()
              n374 = local write "Error 1"(w678) -> ()
              n375 = local write "OFF 1"(TRUE ("OFF 1")) -> ()
              n376 = local write "Ready 1"(w678) -> ()
              n377 = local write "ON 1"(w678) -> ()
            }
            frame 3 {
              w681 = FALSE ("Fault 1")
              n378 = local write "Forming 1"(FALSE ("Forming 1")) -> ()
              n379 = local write "Fault 1"(w681) -> ()
              n380 = local write "Error 1"(w681) -> ()
              n381 = local write "OFF 1"(w681) -> ()
              n382 = local write "Ready 1"(TRUE ("Ready 1")) -> ()
              n383 = local write "ON 1"(w681) -> ()
            }
            frame 4 {
              w684 = FALSE ("Fault 1")
              n384 = local write "Fault 1"(w684) -> ()
              n385 = local write "Error 1"(w684) -> ()
              n386 = local write "OFF 1"(w684) -> ()
              n387 = local write "Ready 1"(w684) -> ()
              n388 = local write "Forming 1"(FALSE ("Forming 1")) -> ()
              n389 = local write "ON 1"(TRUE ("ON 1")) -> ()
            }
            frame 99, Default {
              w686 = FALSE ("Fault 1")
              n390 = local write "Forming 1"(FALSE ("Forming 1")) -> ()
              n391 = local write "Fault 1"(w686) -> ()
              n392 = local write "Error 1"(w686) -> ()
              n393 = local write "OFF 1"(w686) -> ()
              n394 = local write "Ready 1"(w686) -> ()
              n395 = local write "ON 1"(w686) -> ()
            }
          }
          n396 = Bundle By Name(cluster=w665, "State 1"=w658, "code 1"=w659) -> (w664:T6)
        }
        frame 41 {
          w687 = 1.0 ("factor 1")
          n397 = call "U8arrayToMeasurement.vi"("factor 2"=w687, "factor 1"=w687, "payload"=w691) -> ("Meas 2"=w690:dbl)  [unwired: 1 out]
          "V slider 20" <- w690
          n398 = Index Array(array=w691, index=0) -> (element=w697:u8)
          n399 = Index Array(array=w691, index=1) -> (element=w694:u8)
          n400 = Index Array(array=w691, index=2) -> (element=w693:u8)
          n401 = Join Numbers(hi=w694, lo=w693) -> ((hi.lo)=w692:u16)
          "State code 2" <- w692
          n402 = Bundle By Name(cluster=w688, "Vdc2"=w690) -> (w689:T4)
          n403 = case shown="5" w697 {
            frame 5 {
              w702 = FALSE ("Fault 1")
              n404 = local write "Fault 2"(TRUE ("Fault 1")) -> ()
              n405 = local write "Error 2"(w702) -> ()
              n406 = local write "OFF 2"(w702) -> ()
              n407 = local write "Ready 2"(w702) -> ()
              n408 = local write "ON 2"(w702) -> ()
            }
            frame 1 {
              w703 = FALSE ("Fault 1")
              n409 = local write "Fault 2"(w703) -> ()
              n410 = local write "Error 2"(TRUE ("Error 1")) -> ()
              n411 = local write "OFF 2"(w703) -> ()
              n412 = local write "Ready 2"(w703) -> ()
              n413 = local write "ON 2"(w703) -> ()
            }
            frame 2 {
              w706 = FALSE ("Fault 1")
              n414 = local write "Fault 2"(w706) -> ()
              n415 = local write "Error 2"(w706) -> ()
              n416 = local write "OFF 2"(TRUE ("OFF 1")) -> ()
              n417 = local write "Ready 2"(w706) -> ()
              n418 = local write "ON 2"(w706) -> ()
            }
            frame 3 {
              w708 = FALSE ("Fault 1")
              n419 = local write "Fault 2"(w708) -> ()
              n420 = local write "Error 2"(w708) -> ()
              n421 = local write "OFF 2"(w708) -> ()
              n422 = local write "Ready 2"(TRUE ("Ready 1")) -> ()
              n423 = local write "ON 2"(w708) -> ()
            }
            frame 4 {
              w710 = FALSE ("Fault 1")
              n424 = local write "Fault 2"(w710) -> ()
              n425 = local write "Error 2"(w710) -> ()
              n426 = local write "OFF 2"(w710) -> ()
              n427 = local write "Ready 2"(w710) -> ()
              n428 = local write "ON 2"(TRUE ("ON 1")) -> ()
            }
            frame 99, Default {
              w711 = FALSE ("Fault 1")
              n429 = local write "Fault 2"(w711) -> ()
              n430 = local write "Error 2"(w711) -> ()
              n431 = local write "OFF 2"(w711) -> ()
              n432 = local write "Ready 2"(w711) -> ()
              n433 = local write "ON 2"(w711) -> ()
            }
          }
          n434 = Bundle By Name(cluster=w699, "State 2"=w697, "code 2"=w692) -> (w698:T6)
        }
        frame 57 {
          w712 = 1.0 ("factor 1")
          n435 = Index Array(array=w716, index=0) -> (element=w722:u8)
          n436 = Index Array(array=w716, index=1) -> (element=w719:u8)
          n437 = Index Array(array=w716, index=2) -> (element=w718:u8)
          n438 = call "U8arrayToMeasurement.vi"("factor 2"=w712, "factor 1"=w712, "payload"=w716) -> ("Meas 2"=w715:dbl)  [unwired: 1 out]
          "V slider 21" <- w715
          n439 = Join Numbers(hi=w719, lo=w718) -> ((hi.lo)=w717:u16)
          "State code 3" <- w717
          n440 = case shown="5" w722 {
            frame 5 {
              w727 = FALSE ("Fault 1")
              n441 = local write "Fault 3"(TRUE ("Fault 1")) -> ()
              n442 = local write "Error 3"(w727) -> ()
              n443 = local write "OFF 3"(w727) -> ()
              n444 = local write "Ready 3"(w727) -> ()
              n445 = local write "ON 3"(w727) -> ()
            }
            frame 1 {
              w728 = FALSE ("Fault 1")
              n446 = local write "Fault 3"(w728) -> ()
              n447 = local write "Error 3"(TRUE ("Error 1")) -> ()
              n448 = local write "OFF 3"(w728) -> ()
              n449 = local write "Ready 3"(w728) -> ()
              n450 = local write "ON 3"(w728) -> ()
            }
            frame 2 {
              w731 = FALSE ("Fault 1")
              n451 = local write "Fault 3"(w731) -> ()
              n452 = local write "Error 3"(w731) -> ()
              n453 = local write "OFF 3"(TRUE ("OFF 1")) -> ()
              n454 = local write "Ready 3"(w731) -> ()
              n455 = local write "ON 3"(w731) -> ()
            }
            frame 3 {
              w733 = FALSE ("Fault 1")
              n456 = local write "Fault 3"(w733) -> ()
              n457 = local write "Error 3"(w733) -> ()
              n458 = local write "OFF 3"(w733) -> ()
              n459 = local write "Ready 3"(TRUE ("Ready 1")) -> ()
              n460 = local write "ON 3"(w733) -> ()
            }
            frame 4 {
              w735 = FALSE ("Fault 1")
              n461 = local write "Fault 3"(w735) -> ()
              n462 = local write "Error 3"(w735) -> ()
              n463 = local write "OFF 3"(w735) -> ()
              n464 = local write "Ready 3"(w735) -> ()
              n465 = local write "ON 3"(TRUE ("ON 1")) -> ()
            }
            frame 99, Default {
              w736 = FALSE ("Fault 1")
              n466 = local write "Fault 3"(w736) -> ()
              n467 = local write "Error 3"(w736) -> ()
              n468 = local write "OFF 3"(w736) -> ()
              n469 = local write "Ready 3"(w736) -> ()
              n470 = local write "ON 3"(w736) -> ()
            }
          }
          n471 = Bundle By Name(cluster=w713, "Vdc3"=w715) -> (w714:T4)
          n472 = Bundle By Name(cluster=w724, "State 3"=w722, "code 3"=w717) -> (w723:T6)
        }
        frame 73 {
          w737 = 1.0 ("factor 1")
          n473 = Index Array(array=w741, index=0) -> (element=w747:u8)
          n474 = Index Array(array=w741, index=1) -> (element=w744:u8)
          n475 = Index Array(array=w741, index=2) -> (element=w743:u8)
          n476 = Join Numbers(hi=w744, lo=w743) -> ((hi.lo)=w742:u16)
          "State code 4" <- w742
          n477 = call "U8arrayToMeasurement.vi"("factor 2"=w737, "factor 1"=w737, "payload"=w741) -> ("Meas 2"=w738:dbl)  [unwired: 1 out]
          "V slider 22" <- w738
          n478 = case shown="5" w747 {
            frame 5 {
              w752 = FALSE ("Fault 1")
              n479 = local write "Fault 4"(TRUE ("Fault 1")) -> ()
              n480 = local write "Error 4"(w752) -> ()
              n481 = local write "OFF 4"(w752) -> ()
              n482 = local write "Ready 4"(w752) -> ()
              n483 = local write "ON 4"(w752) -> ()
            }
            frame 1 {
              w753 = FALSE ("Fault 1")
              n484 = local write "Fault 4"(w753) -> ()
              n485 = local write "Error 4"(TRUE ("Error 1")) -> ()
              n486 = local write "OFF 4"(w753) -> ()
              n487 = local write "Ready 4"(w753) -> ()
              n488 = local write "ON 4"(w753) -> ()
            }
            frame 2 {
              w756 = FALSE ("Fault 1")
              n489 = local write "Fault 4"(w756) -> ()
              n490 = local write "Error 4"(w756) -> ()
              n491 = local write "OFF 4"(TRUE ("OFF 1")) -> ()
              n492 = local write "Ready 4"(w756) -> ()
              n493 = local write "ON 4"(w756) -> ()
            }
            frame 3 {
              w758 = FALSE ("Fault 1")
              n494 = local write "Fault 4"(w758) -> ()
              n495 = local write "Error 4"(w758) -> ()
              n496 = local write "OFF 4"(w758) -> ()
              n497 = local write "Ready 4"(TRUE ("Ready 1")) -> ()
              n498 = local write "ON 4"(w758) -> ()
            }
            frame 4 {
              w760 = FALSE ("Fault 1")
              n499 = local write "Fault 4"(w760) -> ()
              n500 = local write "Error 4"(w760) -> ()
              n501 = local write "OFF 4"(w760) -> ()
              n502 = local write "Ready 4"(w760) -> ()
              n503 = local write "ON 4"(TRUE ("ON 1")) -> ()
            }
            frame 99, Default {
              w761 = FALSE ("Fault 1")
              n504 = local write "Fault 4"(w761) -> ()
              n505 = local write "Error 4"(w761) -> ()
              n506 = local write "OFF 4"(w761) -> ()
              n507 = local write "Ready 4"(w761) -> ()
              n508 = local write "ON 4"(w761) -> ()
            }
          }
          n509 = Bundle By Name(cluster=w739, "Vdc4"=w738) -> (w740:T4)
          n510 = Bundle By Name(cluster=w749, "State 4"=w747, "code 4"=w742) -> (w748:T6)
        }
        frame 258 {
          w767 = 1000.0 ("factor 1")
          # "Q"
          # "P"
          n511 = call "U8arrayToMeasurement.vi"("factor 2"=w767, "factor 1"=w767, "payload"=w768) -> ("Meas 2"=w762:dbl, "Meas 1"=w763:dbl)
          "kW" <- w763
          "?VkVAr" <- w762
          n512 = Bundle By Name(cluster=w764, "P1"=w763, "Q1"=w762) -> (w765:T4)
        }
        frame 514 {
          w774 = 1000.0 ("factor 1")
          # "Q"
          # "P"
          n513 = call "U8arrayToMeasurement.vi"("factor 2"=w774, "factor 1"=w774, "payload"=w775) -> ("Meas 2"=w771:dbl, "Meas 1"=w772:dbl)
          "kW" <- w772
          "?VkVAr" <- w771
          n514 = Bundle By Name(cluster=w769, "P2"=w772, "Q2"=w771) -> (w770:T4)
        }
        frame 770 {
          w781 = 1000.0 ("factor 1")
          # "Q"
          # "P"
          n515 = call "U8arrayToMeasurement.vi"("factor 2"=w781, "factor 1"=w781, "payload"=w782) -> ("Meas 2"=w778:dbl, "Meas 1"=w779:dbl)
          "kW" <- w779
          "?VkVAr" <- w778
          n516 = Bundle By Name(cluster=w776, "P3"=w779, "Q3"=w778) -> (w777:T4)
        }
        frame 1026 {
          w788 = 1000.0 ("factor 1")
          # "Q"
          # "P"
          n517 = call "U8arrayToMeasurement.vi"("factor 2"=w788, "factor 1"=w788, "payload"=w789) -> ("Meas 2"=w785:dbl, "Meas 1"=w786:dbl)
          "kW" <- w786
          "?VkVAr" <- w785
          n518 = Bundle By Name(cluster=w783, "P4"=w786, "Q4"=w785) -> (w784:T4)
        }
        frame 262 {
          w795 = 1.0 ("factor 1")
          n519 = call "U8arrayToMeasurement.vi"("factor 2"=w795, "factor 1"=w795, "payload"=w794) -> ("Meas 1"=w793:dbl)  [unwired: 1 out]
          n520 = Bundle By Name(cluster=w790, "Vdc1"=w793) -> (w791:T4)
        }
        frame 518 {
          w803 = 1.0 ("factor 1")
          # "Vdc"
          n521 = call "U8arrayToMeasurement.vi"("factor 2"=w803, "factor 1"=w803, "payload"=w802) -> ("Meas 2"=w800:dbl, "Meas 1"=w801:dbl)
          n522 = Add(x=w801, y=w800) -> (x+y=w799:dbl)
          n523 = Bundle By Name(cluster=w797, "Vdc2"=w799) -> (w796:T4)
        }
        frame 774 {
          w811 = 1.0 ("factor 1")
          # "Vdc"
          n524 = call "U8arrayToMeasurement.vi"("factor 2"=w811, "factor 1"=w811, "payload"=w810) -> ("Meas 2"=w808:dbl, "Meas 1"=w809:dbl)
          n525 = Add(x=w809, y=w808) -> (x+y=w804:dbl)
          n526 = Bundle By Name(cluster=w806, "Vdc3"=w804) -> (w805:T4)
        }
        frame 1030 {
          w819 = 1.0 ("factor 1")
          # "Vdc"
          n527 = call "U8arrayToMeasurement.vi"("factor 2"=w819, "factor 1"=w819, "payload"=w818) -> ("Meas 2"=w816:dbl, "Meas 1"=w817:dbl)
          n528 = Add(x=w817, y=w816) -> (x+y=w812:dbl)
          n529 = Bundle By Name(cluster=w813, "Vdc4"=w812) -> (w814:T4)
        }
      }
      n530 = local write "measurements"(w644) -> ()
      n531 = local write "conv"(w646) -> ()
      "CAN IN" <- w648
    }
    n532 = local read "main stop"() -> (w640:bool)
    n533 = node-c288() -> ()  [unwired: 1 in, 1 out]
  }
  n534 = call <instrlib>:"niSync Close.vi"("error in (no error)"=w20, "instrument handle"=w21) -> ("error out"=→"Error out":errorcluster)  [unwired: 9 in]
  n535 = UDP Close(connection ID=w1, 8:w6) -> ()  [unwired: 2 out]
  n536 = while {
    stop <- w822 stop-if-true
    n537 = flat-sequence {
      tunnel: [w824] -> w823
      tunnel: w823 -> [w831]
      frame #0 {
        n538 = local read "start following 1 pre"() -> (w825:bool)
        n539 = call <userlib>:"Boolean Trigger__ogtk.vi"("Boolean Input"=w825) -> ("Rising Edge"=w826:bool)  [unwired: 1 in, 1 out]
        n540 = case shown="True" w826 {
          tunnel: w825 -> [w827 w828]
          tunnel: [w827 w828] -> w824
          frame False {
          }
          frame True {
            n541 = Get Date/Time In Seconds() -> (seconds since 1Jan1904=→"time_afe":timestamp)
            n542 = Wait (ms)(milliseconds to wait=u32 550) -> ()  [unwired: 1 out]
          }
        }
      }
      frame #1 {
        n543 = local write "Start following 1"(w831) -> ()
      }
    }
    n544 = local read "main stop"() -> (w822:bool)
  }
  n545 = node-c288(w42) -> ()  [unwired: 1 out]
  n546 = node-c288(w37) -> ()  [unwired: 1 out]
  n547 = call <vilib>:"XNET Stop.vi"("session in"=w47) -> ()  [unwired: 13 in, 2 out]
  n548 = local write "CAN with Conv"(w45) -> ()
  n549 = call <vilib>:"XNET Stop.vi"("session in"=w48) -> ()  [unwired: 13 in, 2 out]
  n550 = UDP Close(connection ID=w10, 8:w9) -> ()  [unwired: 2 out]
  "Measurements" <- w34
  "CAN with Conv" <- w34
  "logging" <- w34
  "Ready 1" <- w34
  "OFF 1" <- w34
  "Ready 2" <- w34
  "ON 2" <- w34
  "OFF 2" <- w34
  "Ready 4" <- w34
  "ON 4" <- w34
  "OFF 4" <- w34
  "ON 3" <- w34
  "Ready 3" <- w34
  "OFF 3" <- w34
  "Fault 1" <- w34
  "Error 1" <- w34
  "Fault 2" <- w34
  "Error 2" <- w34
  "Fault 3" <- w34
  "Error 3" <- w34
  "Fault 4" <- w34
  "Error 4" <- w34
  "Forming 2" <- w28
  "Forming 1" <- w28
